vi "校准UI.vi"() -> ()   [LabVIEW 2016, in "斯坦道多参数.lvlib"]
uses:
  <vilib>/Utility/miscctls.llb/LVPointTypeDef.ctl
  <vilib>/Utility/miscctls.llb/LVPositionTypeDef.ctl
  <vilib>/ptbypt/NI_PtbyPt.lvlib
panel:
  out "溶解氧浓度值":dbl=25.0 caption="检测值：" format="%#.2f mg/L"
  out "电极状态标志":u16
  in  "恢复出厂":bool
  in  "电极系数面板":enum32{"选项卡 1"}(tab)
  out "B":dbl=25.0 caption="电极零点：" format="%#.6f"
  out "K":dbl=25.0 caption="电极系数：" format="%#.6f"
  in  "测试参数面板":enum32{"选项卡 1"}(tab)
  in  "自动盐度补偿":bool caption="自动盐度补偿："
  in  "偏移修正值":dbl=25.0 caption="偏移修正值：" format="%#_6f"
  in  "滤波次数":dbl=25.0 caption="滤波次数：" format="%#_6f"
  in  "测量量程":u16(ring)=1 caption="测量量程："
  in  "盐度":dbl=25.0 caption="盐度：" format="%#_6f"
  in  "大气压力":dbl=25.0 caption="大气压力：" format="%#_6f"
  in  "温度系数":dbl=25.0 caption="温度系数：" format="%#6.f"
  out "信号值":dbl=25.0 caption="信号值：" format="%#.2f"
  out "检测值":dbl=25.0 caption="检测值：" format="%#.2f"
  out "序列号":string caption="序列号："
  in  "选项卡控件 3":enum32{"选项卡 1"}(tab)
  in  "清扫间隔":u16=25 caption="清扫间隔："
  in  "清扫次数":u16=25 caption="清扫次数："
  in  "清洗":bool caption="探头清洗："
  in  "清扫模式":u16(ring)=1 caption="清扫模式：" items=["自动", "手动"]
  in  "选项卡控件 2":enum32{"选项卡 1"}(tab)
  in  "实际温度":dbl=25.0 caption="实际温度：" format="%.2f ℃"
  out "当前温度":dbl caption="当前温度：" format="%.2f ℃"
  in  "校准温度":bool
  in  "选项卡控件":enum32{"选项卡 1"}(tab)
  in  "第三点确认校准":bool
  in  "第二点确认校准":bool
  in  "标液一":cluster{"标准值":dbl, "检测值":dbl, "原始值":dbl} caption="标液一：" {"原始值" format="%#_6f"; "检测值" format="%#_6f"; "标准值" format="%#.6f"}
  in  "标液二":cluster{"标准值":dbl, "检测值":dbl, "原始值":dbl} caption="标液二：" {"原始值" format="%#_6f"; "检测值" format="%#_6f"; "标准值" format="%#.6f"}
  in  "标液三":cluster{"标准值":dbl, "检测值":dbl, "原始值":dbl} caption="标液三：" {"原始值" format="%#_6f"; "检测值" format="%#_6f"; "标准值" format="%#.6f"}
  in  "标液一开始校准":bool
  in  "第一点确认校准":bool
  in  "标液二开始校准":bool
  in  "标液三开始校准":bool
  in  "显示曲线":bool
  in  "校准记录":string="校准记录\n---------------------------------------------\n序列号：\n温度值：\n标准值：\n检测值：\n原始值：\n校准时间："
  in  "校准方式":u16(ring)=1 caption="校准方式：" items=["单点校准", "两点校准", "三点校准"]
  in  "校准参数":u16(ring) caption="校准参数：" items=["pH", "DO", "浊度", "电导率"]
  # "检测值"
  # "信号值"
  # "标准值"
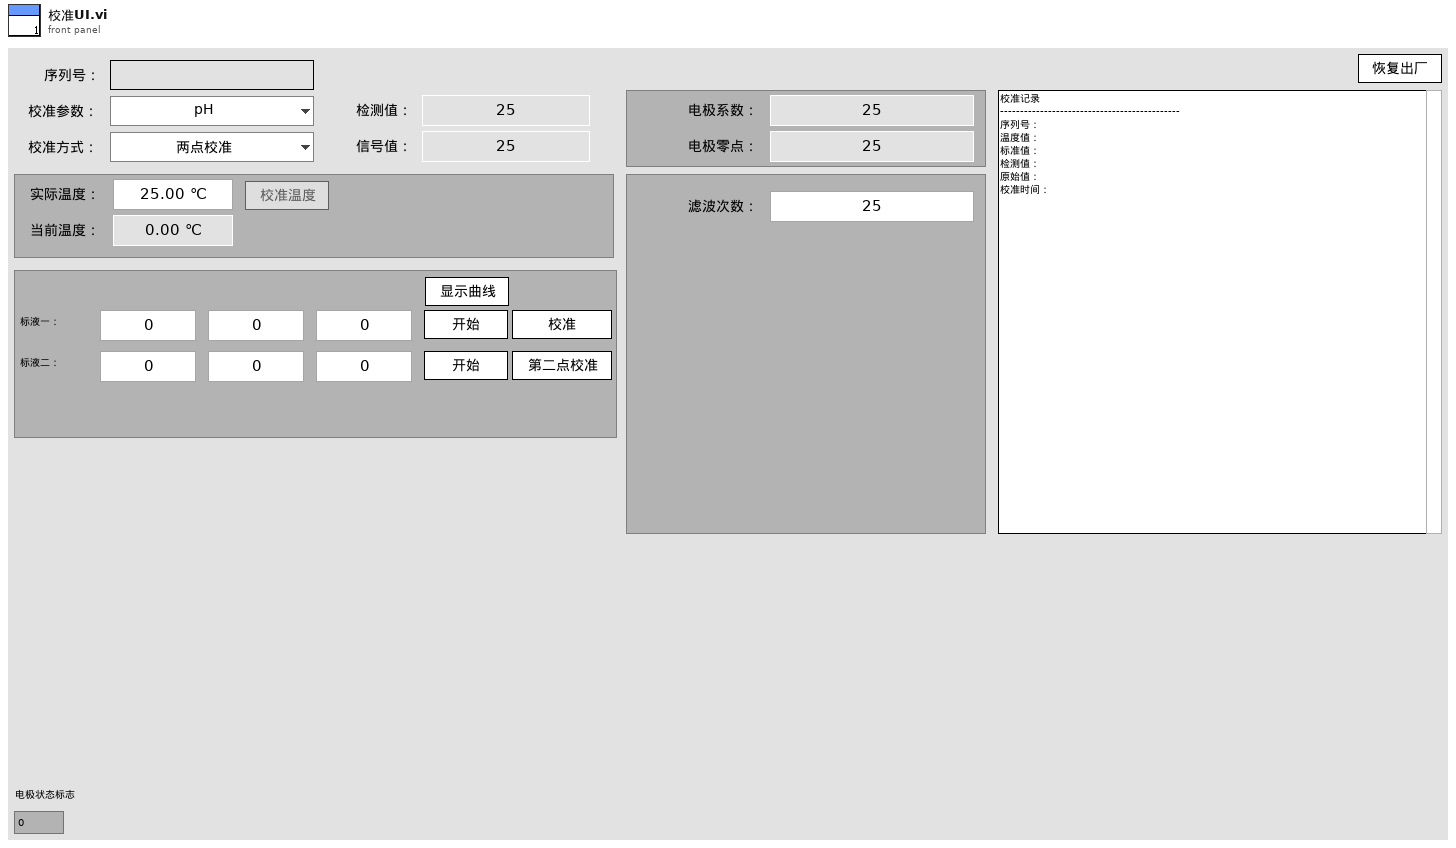
[diagram p1: front panel]
types:
  T1 = typedef "LVPointTypeDef.ctl" = cluster{"Horizontal":i16, "Vertical":i16}
  T2 = cluster{"ph":bool, "DO":bool, "Cond":bool, "Turb":bool, "叶绿素a":bool, "藻密度":bool, "ORP":bool, "COD":bool, "DO2":bool}
  T3 = typedef "LVStringsAndValuesArrayTypeDef_U16.ctl" = cluster{"String":string, "Value":u16}[]
  T4 = enum8{"Enabled", "Disabled", "Disabled and Grayed Out"}
  T5 = typedef "LVPositionTypeDef.ctl" = cluster{"Left":i32, "Top":i32}
  T6 = cluster{"pH":u32, "DO":u32, "Cond":u32, "Turb":u32, "叶绿素a":u32, "藻密度":u32, "ORP":u32, "COD":u32}
  T7 = cluster{"电极状态标志":u16, "电极型号标志":u16, "酸碱度测量值":sgl, "温度测量值":sgl, "酸碱度信号值":sgl, "温度信号值":sgl, "酸碱度偏移修正值":sgl, "温度偏移修正值":sgl, "手动温度补偿值":sgl, "酸碱度电极零点":sgl, "酸碱度电极斜率":sgl, "第1点标准值记录":sgl, "第1点信号值记录":sgl, "第1点温度值记录":sgl, "第2点标准值记录":sgl, "第2点信号值记录":sgl, "第2点温度值记录":sgl, "命令滤波设定":u16, "温度模式":enum16{"ATC", "MTC"}, "生产批次":u16, "电极序号":u16, "串口地址":u16, "串口波特率":enum16{"9600", "19200", "115200"}, "串口校验位":enum16{"NONE", "ODD", "EVEN"}, "串口停止位":enum16{"1bit", "2bit"}, "第一点标准值":sgl, "第二点标准值":sgl}
  T8 = cluster{"报警码":u16, "溶解氧数值（mg/L）":sgl, "溶解氧数据（%）":sgl, "温度数据":sgl, "溶解氧原始信号 nA":sgl, "大气压力":sgl, "盐度":sgl, "0X0009_NC":string, "产品名称":string, "序列号":string, "硬件版本":string, "软件版本":string, "通讯地址":u16, "波特率":u16, "设备类型":u16, "0X0026_NC":string, "第一点原始数据":sgl, "第一点校准数据":sgl, "第二点原始数据":sgl, "第二点校准数据":sgl, "探头校准命令":u16, "温度校准参数":sgl, "温度校准命令":u16}
  T9 = cluster{"电极状态标志":u16, "电极型号标志":u16, "溶解氧测量值":sgl, "温度测量值":sgl, "溶解氧饱和度值":sgl, "盐度补偿值":sgl, "大气压补偿值":sgl, "溶解氧偏移修正值":sgl, "温度偏移修正值":sgl, "手动温度补偿值":sgl, "溶解氧电极零点":sgl, "溶解氧电极斜率":sgl, "第1点标准值记录":sgl, "第1点信号值记录":sgl, "第1点温度值记录":sgl, "第2点标准值记录":sgl, "第2点信号值记录":sgl, "第2点温度值记录":sgl, "命令滤波设定":u16, "温度模式":enum16{"ATC", "MTC"}, "生产批次":u16, "电极序号":u16, "串口地址":u16, "串口波特率":enum16{"9600", "19200", "115200"}, "串口校验位":enum16{"NONE", "ODD", "EVEN"}, "串口停止位":enum16{"1bit", "2bit"}, "第一点标准值":sgl, "第二点标准值":sgl}
  T10 = cluster{"电极状态标志":u16, "电极型号标志":u16, "浊度测量值":sgl, "温度测量值":sgl, "浊度信号值":sgl, "浊度偏移修正值":sgl, "温度偏移修正值":sgl, "手动温度补偿值":sgl, "浊度电极零点":sgl, "浊度电极斜率":sgl, "清洁周期":u16, "命令滤波设定":u16, "温度模式":enum16{"ATC", "MTC"}, "生产批次":u16, "电极序号":u16, "串口地址":u16, "串口波特率":enum16{"9600", "19200", "115200"}, "串口校验位":enum16{"NONE", "ODD", "EVEN"}, "串口停止位":enum16{"1bit", "2bit"}, "第一点标准值":sgl, "第二点标准值":sgl, "第三点标准值":sgl}
  T11 = cluster{"报警码":u16, "浊度数值 NTU":sgl, "温度数据":sgl, "原始光强数值":u16, "量程":u16, "平均次数":u16, "清扫模式":u16, "清扫次数":u16, "清扫间隔分钟":u16, "0X000B_NC":string, "产品名称":string, "序列号":string, "硬件版本":string, "软件版本":string, "通讯地址":u16, "波特率":u16, "设备类型":u16, "0X0026_NC":string, "校准量程":u16, "第一点原始光强":u16, "第一点校准数据":sgl, "第二点原始光强":u16, "第二点校准数据":sgl, "第三点原始光强":u16, "第三点校准数据":sgl, "探头校准命令":u16, "温度校准参数":sgl, "温度校准命令":u16}
  T12 = cluster{"电极状态标志":u16, "电极型号标志":u16, "电导率测量值":sgl, "温度测量值":sgl, "电导率信号值":sgl, "温度信号值":sgl, "温度补偿系数":sgl, "电导率偏移修正值":sgl, "温度偏移修正值":sgl, "手动温度补偿值":sgl, "电导率电极零点":sgl, "电导率电极斜率":sgl, "命令滤波设定":u16, "温度模式":enum16{"ATC", "MTC"}, "生产批次":u16, "电极序号":u16, "串口地址":u16, "串口波特率":enum16{"9600", "19200", "115200"}, "串口校验位":enum16{"NONE", "ODD", "EVEN"}, "串口停止位":enum16{"1bit", "2bit"}, "第一点标准值":sgl, "第二点标准值":sgl}
  T13 = cluster{"报警码":u16, "叶绿素a":sgl, "温度数据":sgl, "原始光强数值":u16, "量程":u16, "平均次数":u16, "清扫模式":u16, "清扫次数":u16, "清扫间隔分钟":u16, "0X000B_NC":string, "产品名称":string, "序列号":string, "硬件版本":string, "软件版本":string, "通讯地址":u16, "波特率":u16, "设备类型":u16, "0X0026_NC":string, "校准量程":u16, "第一点原始光强":u16, "第一点校准数据":sgl, "第二点原始光强":u16, "第二点校准数据":sgl, "第三点原始光强":u16, "第三点校准数据":sgl, "探头校准命令":u16, "温度校准参数":sgl, "温度校准命令":u16}
  T14 = cluster{"报警码":u16, "蓝绿藻":sgl, "温度数据":sgl, "原始光强数值":u16, "量程":u16, "平均次数":u16, "清扫模式":u16, "清扫次数":u16, "清扫间隔分钟":u16, "0X000B_NC":string, "产品名称":string, "序列号":string, "硬件版本":string, "软件版本":string, "通讯地址":u16, "波特率":u16, "设备类型":u16, "0X0026_NC":string, "校准量程":u16, "第一点原始光强":u16, "第一点校准数据":sgl, "第二点原始光强":u16, "第二点校准数据":sgl, "第三点原始光强":u16, "第三点校准数据":sgl, "探头校准命令":u16, "温度校准参数":sgl, "温度校准命令":u16}
  T15 = cluster{"电极状态标志":u16, "电极型号标志":u16, "测量值":sgl, "温度测量值":sgl, "信号值":sgl, "温度信号值":sgl, "000AH_NC":sgl, "偏移修正值":sgl, "温度偏移修正值":sgl, "手动温度补偿值":sgl, "命令滤波设定":u16, "温度模式":enum16{"ATC", "MTC"}, "生产批次":u16, "传感器序号":u16, "串口地址":u16, "串口波特率":enum16{"9600", "19200", "115200"}, "串口校验位":enum16{"NONE", "ODD", "EVEN"}, "串口停止位":enum16{"1bit", "2bit"}}
  T16 = enum16{"null", "pH", "DO", "浊度", "电导率", "叶绿素a", "藻密度"}
  T17 = cluster{"禁用":enum8{"Enabled", "Disabled", "Disabled and Grayed Out"}, "禁用 2":enum8{"Enabled", "Disabled", "Disabled and Grayed Out"}, "禁用 3":enum8{"Enabled", "Disabled", "Disabled and Grayed Out"}}
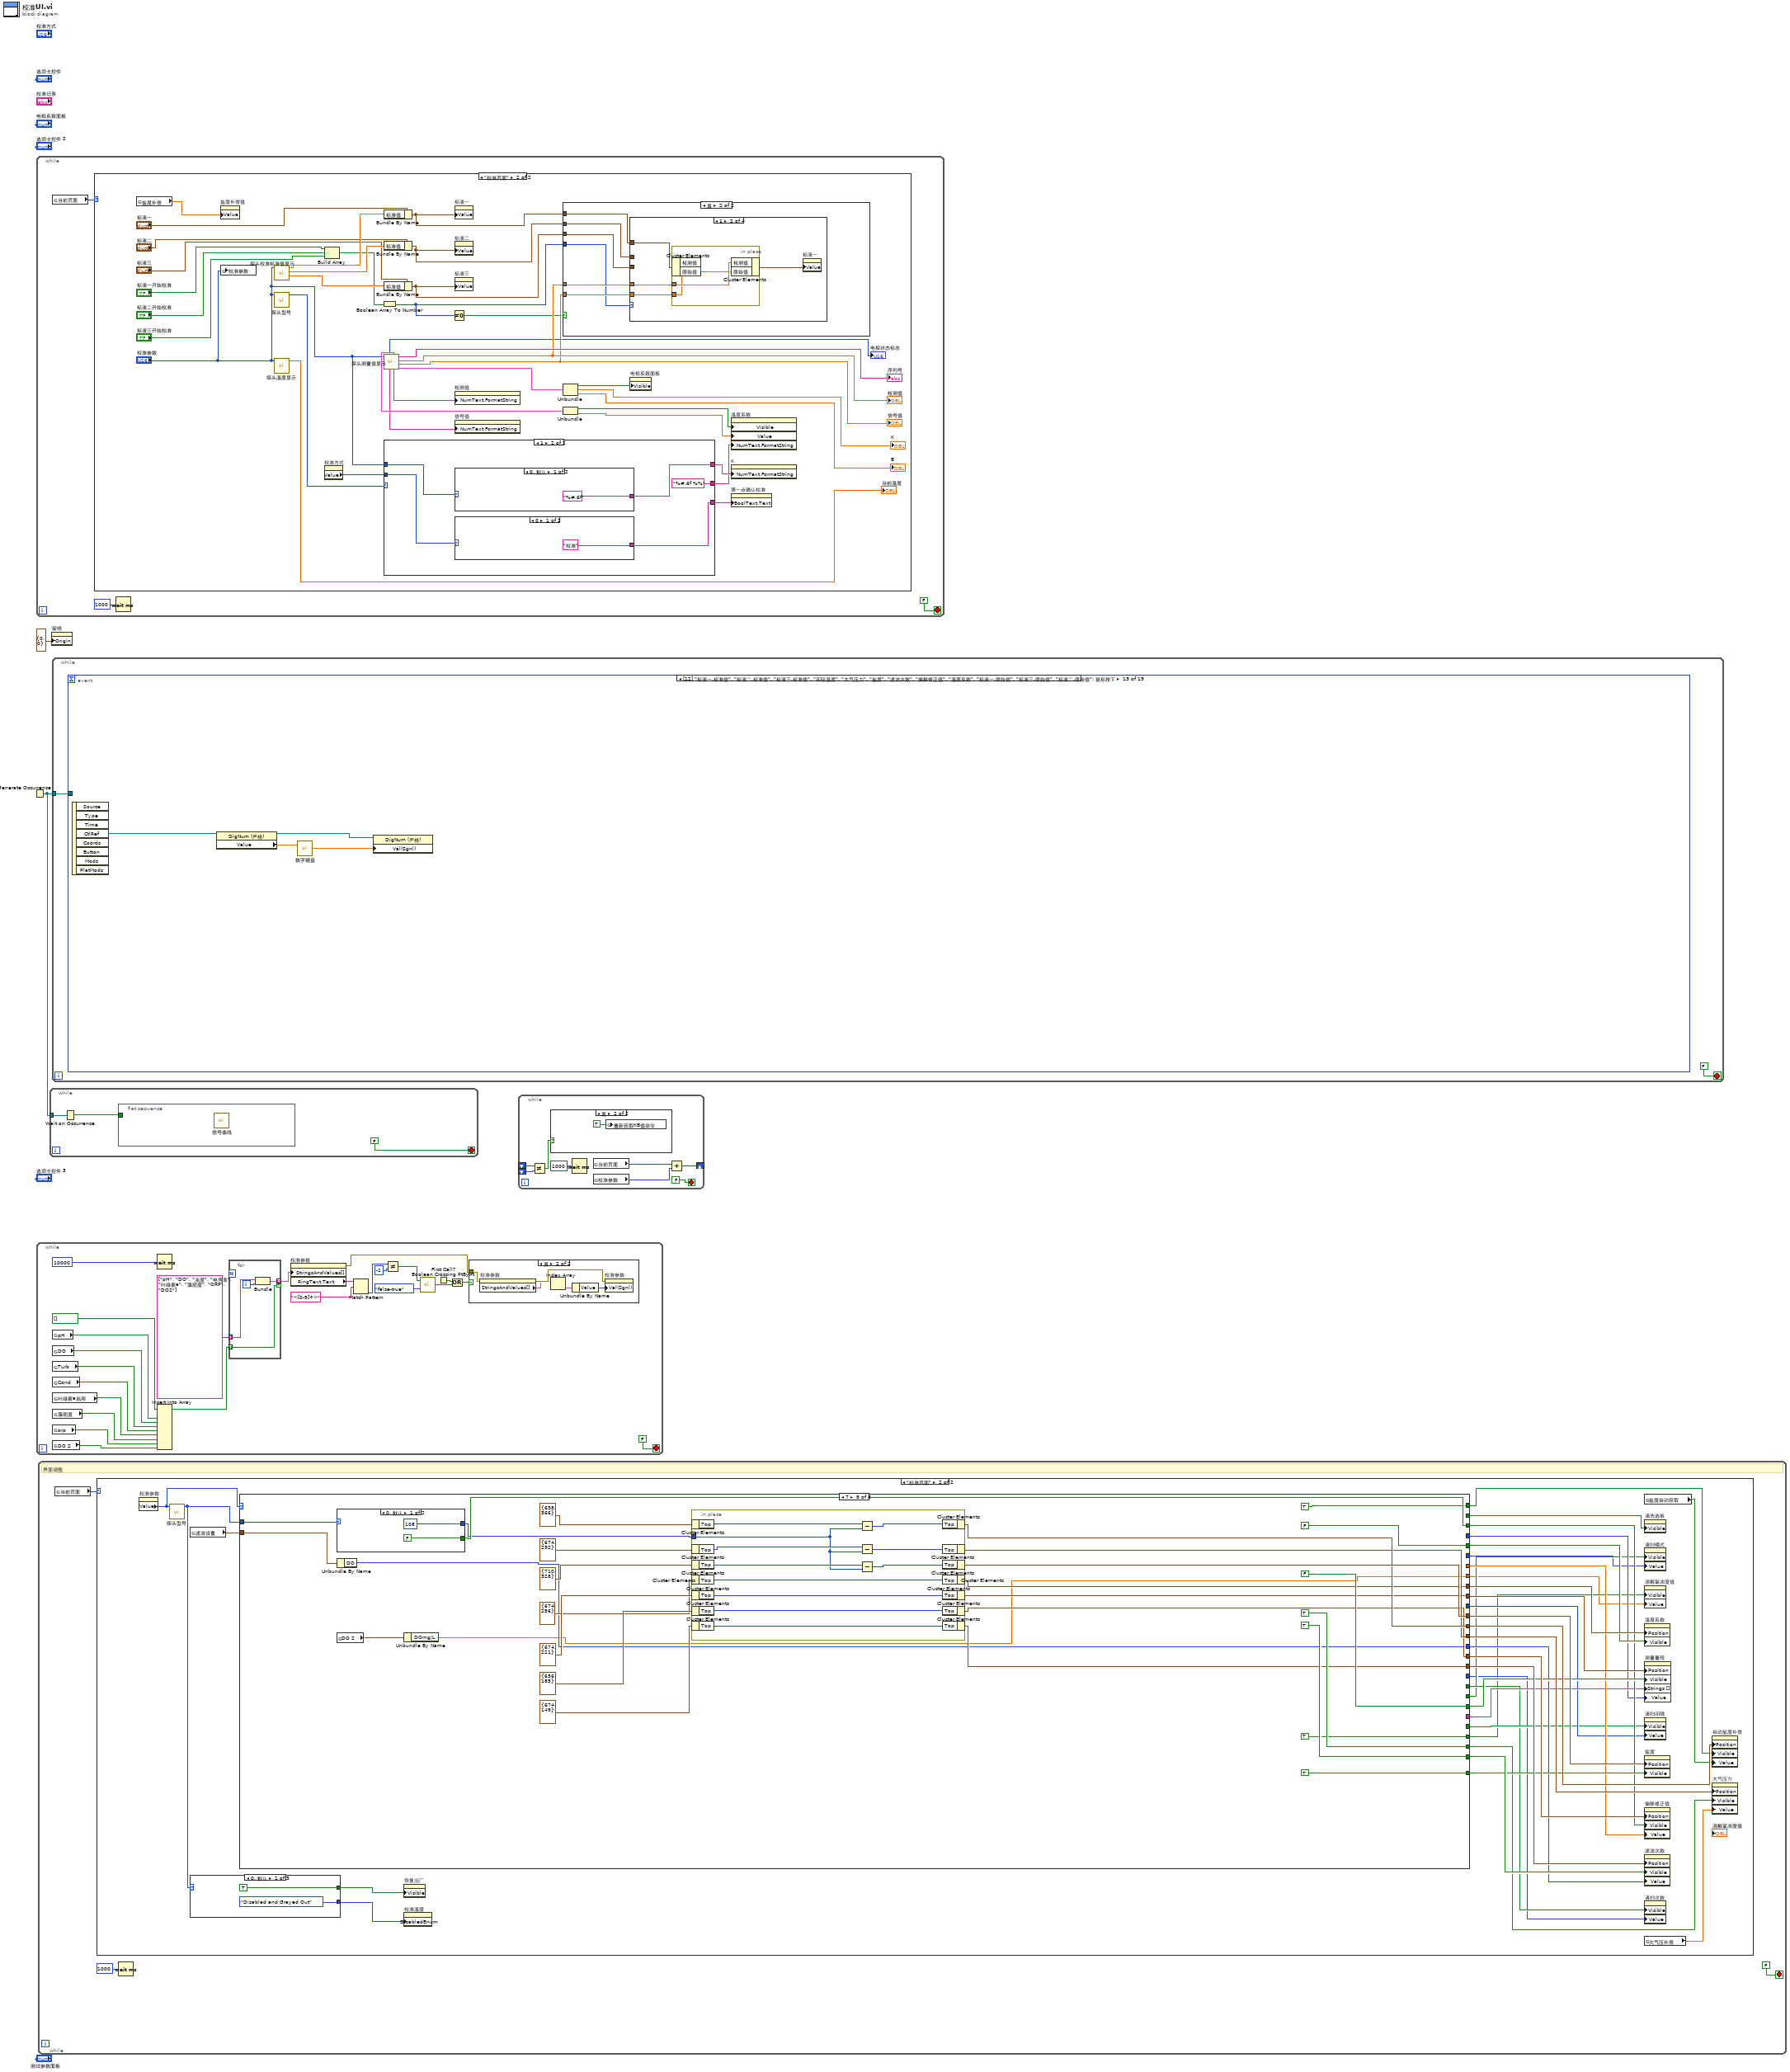
[diagram p0: block diagram]
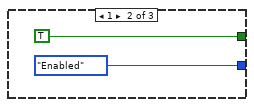
[diagram p4: hidden frame]
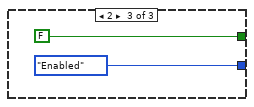
[diagram p5: hidden frame]
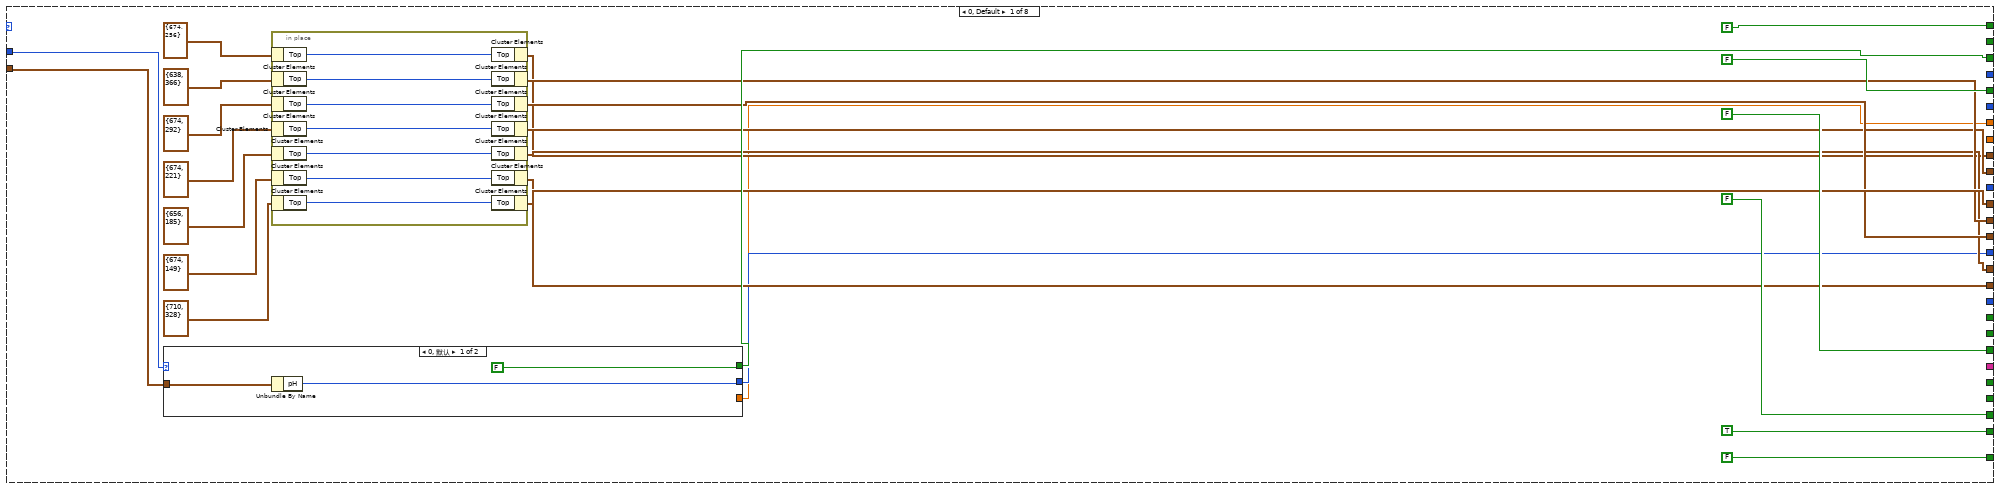
[diagram p6: hidden frame]
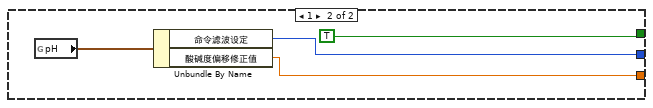
[diagram p7: hidden frame]
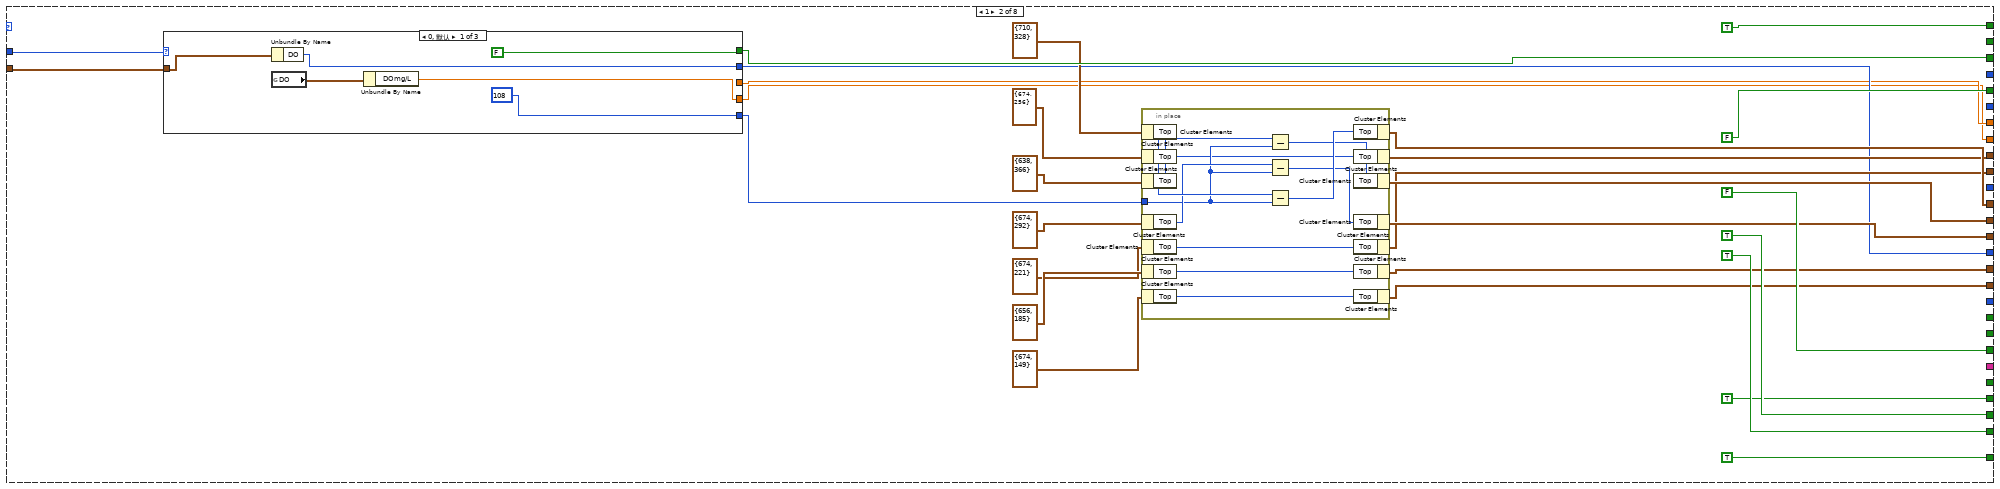
[diagram p8: hidden frame]
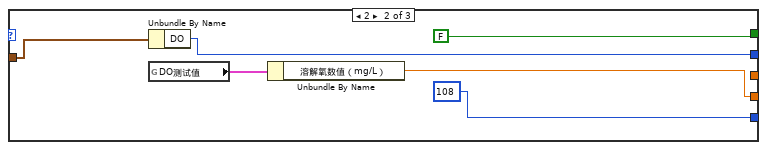
[diagram p9: hidden frame]
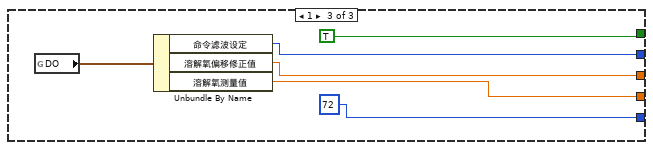
[diagram p10: hidden frame]
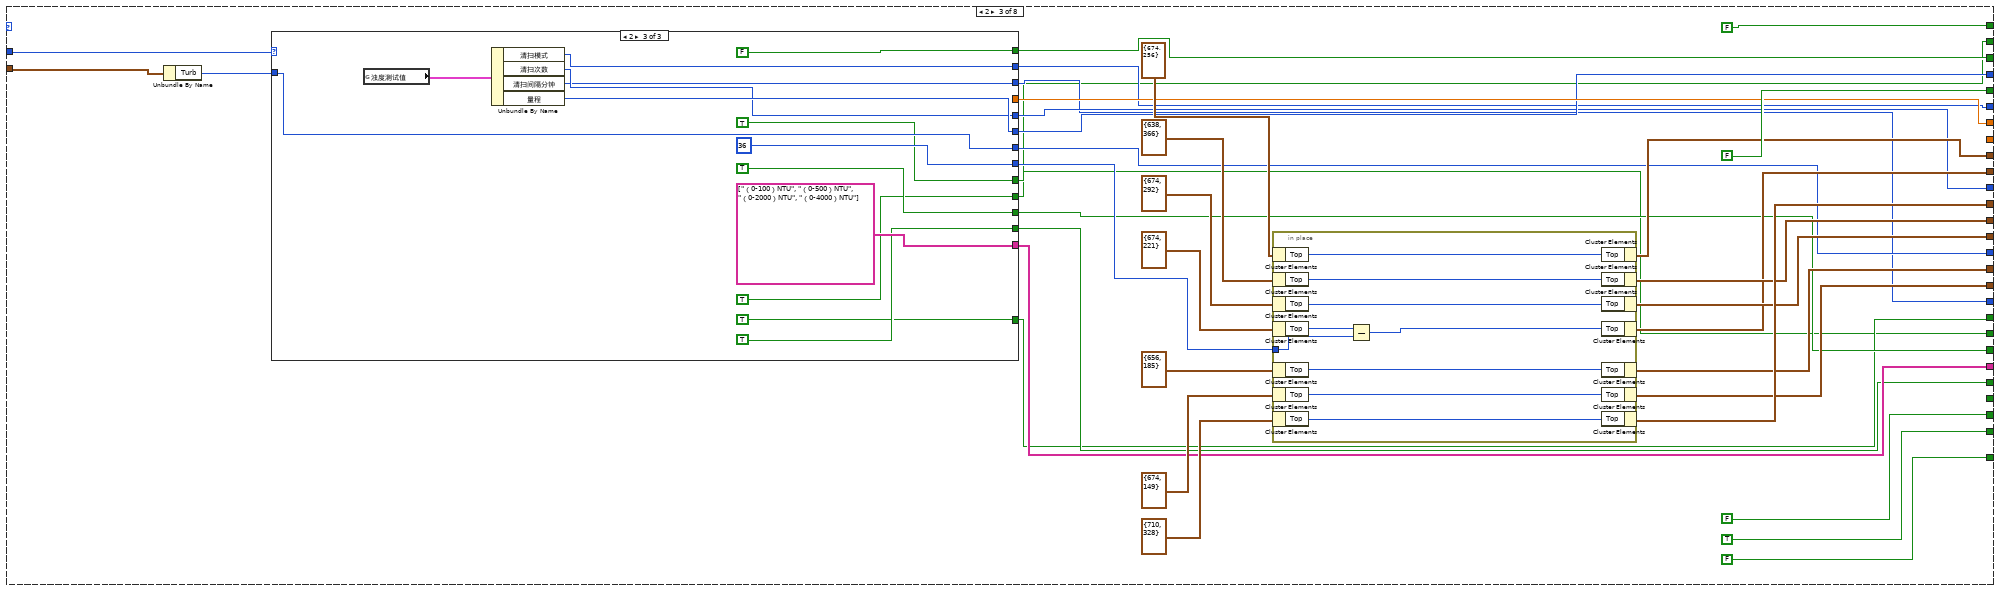
[diagram p11: hidden frame]
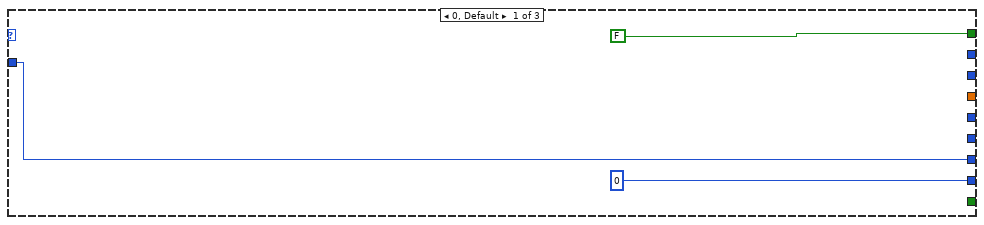
[diagram p12: hidden frame]
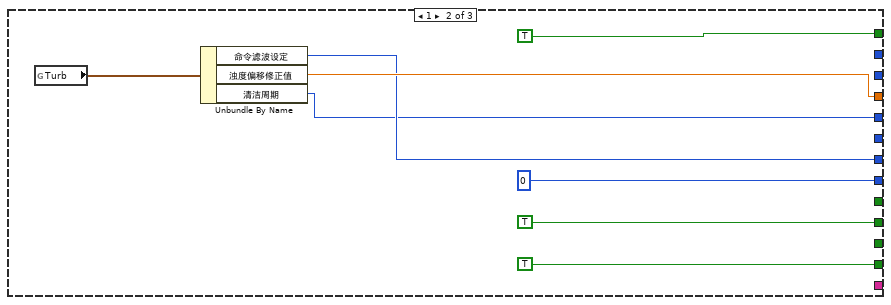
[diagram p13: hidden frame]
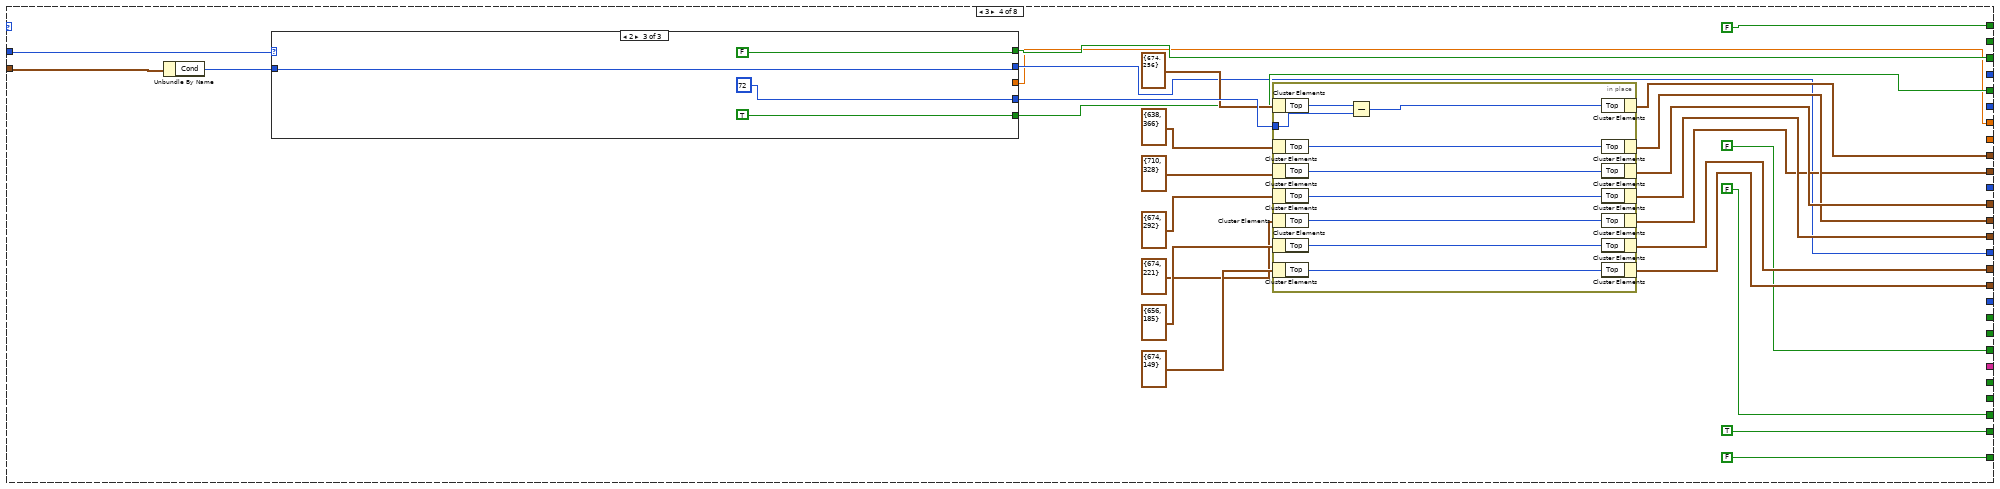
[diagram p14: hidden frame]
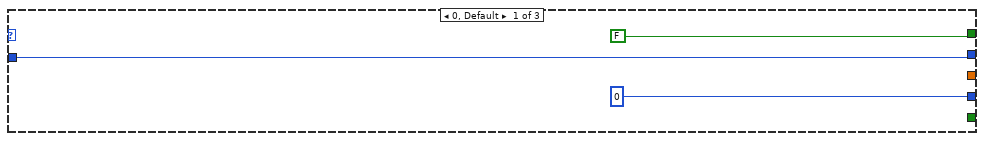
[diagram p15: hidden frame]
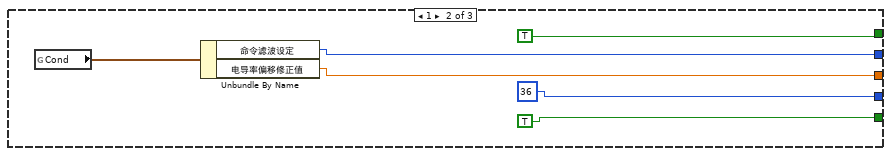
[diagram p16: hidden frame]
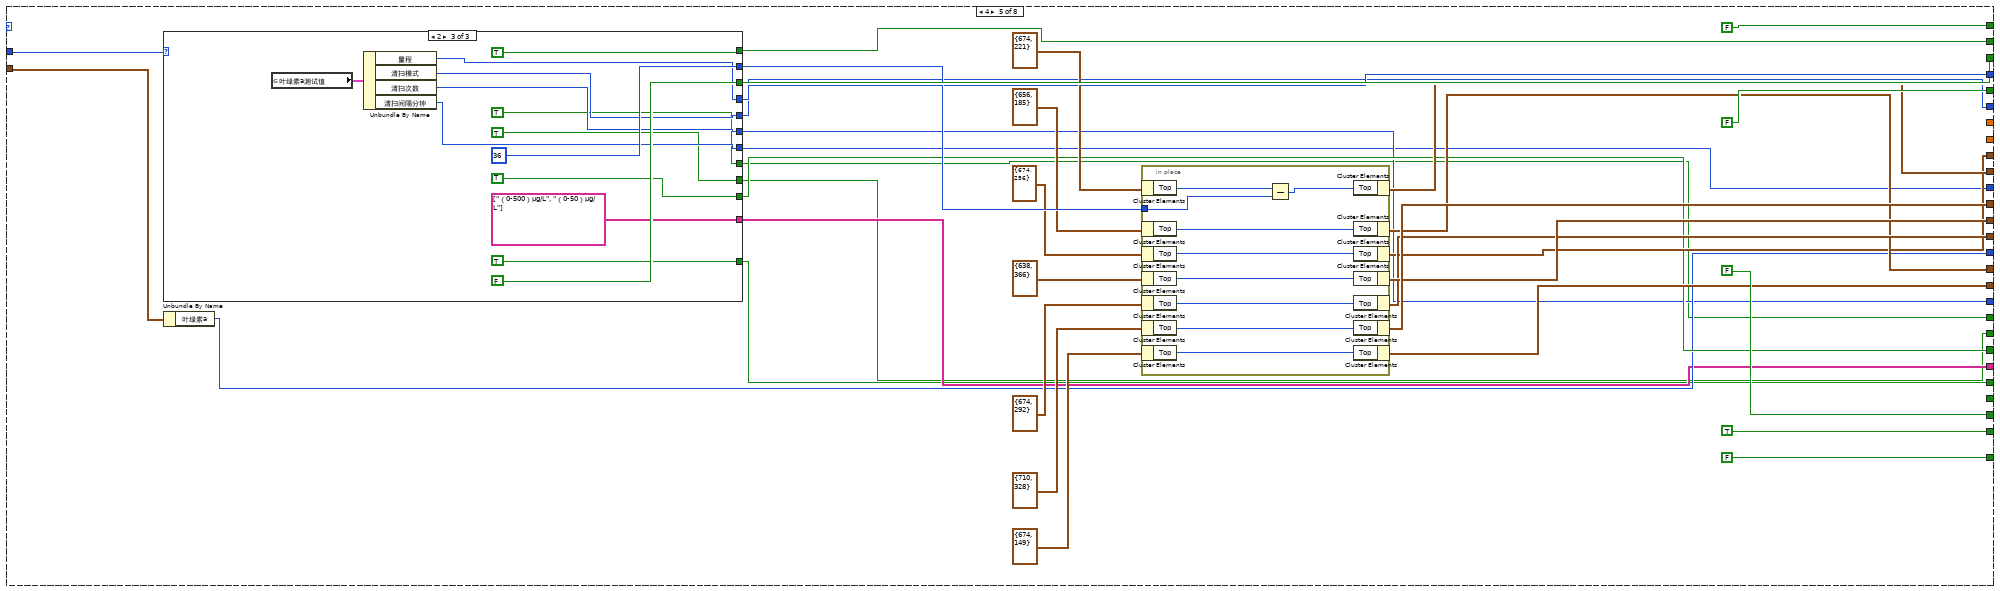
[diagram p17: hidden frame]
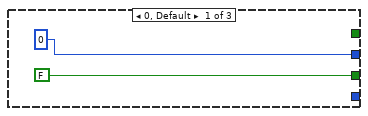
[diagram p18: hidden frame]
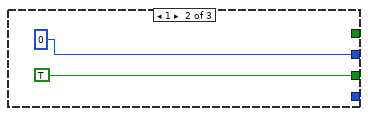
[diagram p19: hidden frame]
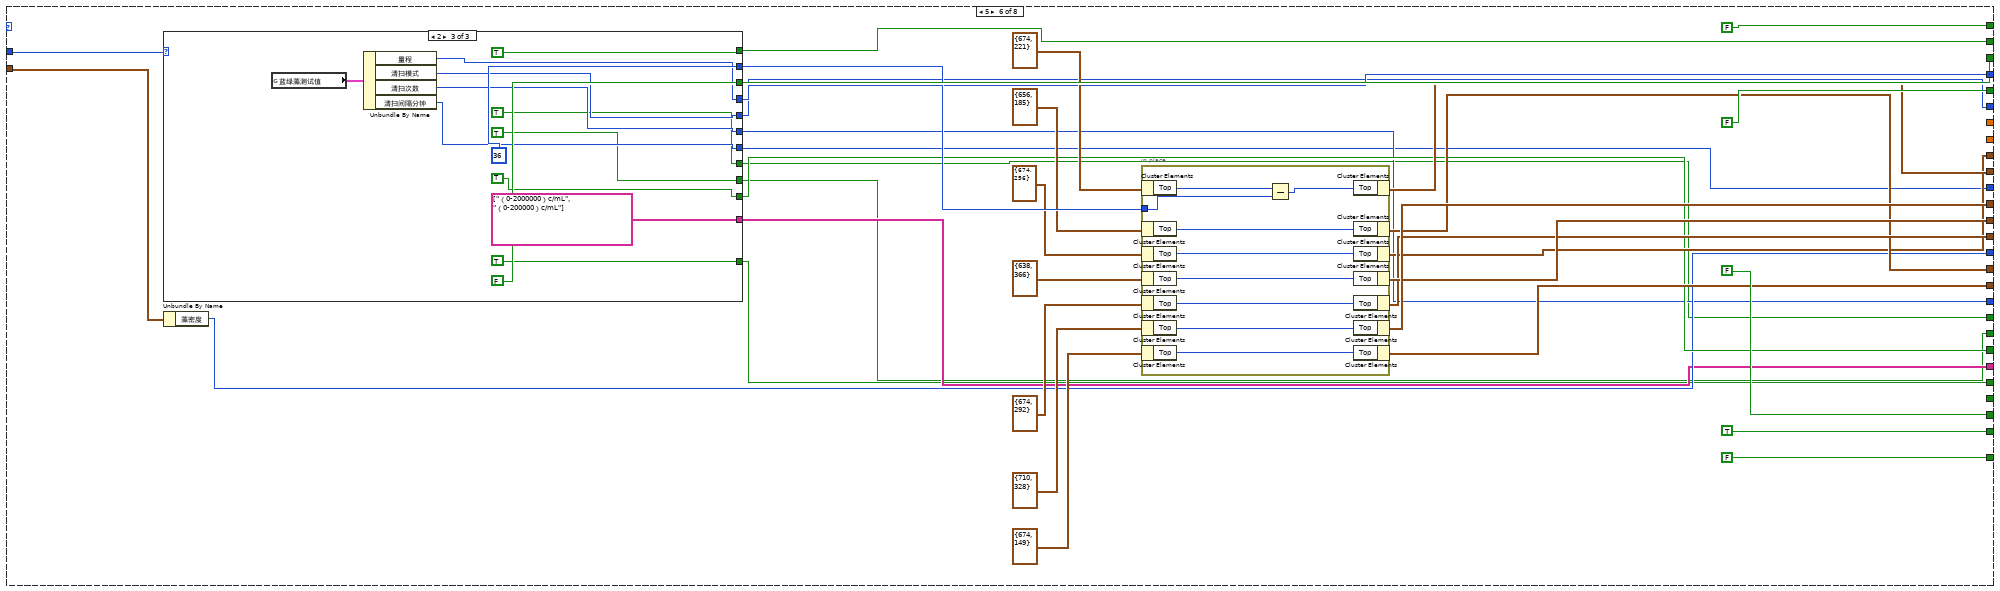
[diagram p20: hidden frame]
diagram:
  n1 = Generate Occurrence() -> (w1:refnum<k4>)
  n2 = while {
    stop <- FALSE stop-if-true
    n3 = global read "多参数全局变量.vi" "当前页面"() -> (w3:enum16{"主页面", "参数页面", "校准页面"})
    n4 = case shown="\"校准页面\"" w3 {
      frame "主页面", Default {
        n5 = global write "多参数全局变量.vi" "校准运行状态"(T2 {"ph"=FALSE, "DO"=FALSE, "Cond"=FALSE, "Turb"=FALSE, "叶绿素a"=FALSE, "藻密度"=FALSE, "ORP"=FALSE, "COD"=FALSE, "DO2"=FALSE} ("校准运行状态")) -> ()
      }
      frame "校准页面" {
        n6 = global read "断电保存变量.vi" "盐度补偿"() -> (w29:dbl)
        n7 = property on="盐度补偿值" class="DigNum (严格)"("Value"=w29) -> ()  [unwired: 2 in, 2 out]
        n8 = global write "多参数全局变量.vi" "校准参数"("校准参数") -> ()
        n9 = call "探头校准标准值显示.vi"("校准参数"="校准参数") -> ("标液三"=w42:sgl, "标液二"=w41:sgl, "标液一"=w40:sgl)  [unwired: 8 in]
        n10 = call "探头型号.vi"("校准参数"="校准参数") -> ("探头型号"=w24:u16)  [unwired: 8 in, 2 out]
        n11 = call "探头温度显示.vi"("校准参数"="校准参数") -> ("温度数据"=→"当前温度":sgl)  [unwired: 9 in, 1 out]
        n12 = Build Array("标液一开始校准", "标液二开始校准", "标液三开始校准") -> (w10:bool[])
        n13 = property on="校准方式" class="Ring (严格)"() -> ("Value"=w22:u16)  [unwired: 2 in, 2 out]
        n14 = Boolean Array To Number(Boolean array=w10) -> (number=w8:u32)
        n15 = Bundle By Name(cluster="标液一", "标准值"=w40) -> (w36:cluster{"标准值":dbl, "检测值":dbl, "原始值":dbl})
        n16 = Bundle By Name(cluster="标液二", "标准值"=w41) -> (w35:cluster{"标准值":dbl, "检测值":dbl, "原始值":dbl})
        n17 = Bundle By Name(cluster="标液三", "标准值"=w42) -> (w34:cluster{"标准值":dbl, "检测值":dbl, "原始值":dbl})
        n18 = call "探头测量值显示.vi"("校准参数"="校准参数") -> ("线性系数"=w28:cluster{bool, "K":sgl, "B":sgl}, "信号值"=w30:sgl, "检测值"=w31:sgl, "序列号"=→"序列号":string, "检测值.格式字符串"=w21:string, "温度补偿系数"=w20:cluster{bool, "温度补偿系数":sgl}, "信号值.格式字符串"=w16:string, "电极状态标志"=→"电极状态标志":u16)  [unwired: 3 in]
        "检测值" <- w31
        "信号值" <- w30
        n19 = case shown="1" w24 {
          tunnel: ["校准" w50] -> w23
          tunnel: w22 -> [_ w49]
          tunnel: "校准参数" -> [_ w48]
          tunnel: ["%#.6f" ("数值文本.格式字符串") w47] -> w15
          tunnel: ["%#.6f" ("数值文本.格式字符串") "%#.6f %%" ("数值文本.格式字符串")] -> w14
          frame 0, Default {
          }
          frame 1 {
            n20 = case shown="0, 默认" w48 {
              tunnel: ["%#.6f" ("数值文本.格式字符串") "%#.6f (1/cm)" ("数值文本.格式字符串")] -> w47
              frame 0, Default {
              }
              frame 3 {
              }
            }
            n21 = case shown="0" w49 {
              tunnel: ["校准" "第一点校准"] -> w50
              frame 0 {
              }
              frame 1, Default {
              }
            }
          }
        }
        n22 = Not Equal To 0?(x=w8) -> (x != 0?=w9:bool)
        n23 = property on="标液一" class="Clust (严格)"("Value"=w36) -> ()  [unwired: 2 in, 2 out]
        n24 = property on="标液二" class="Clust (严格)"("Value"=w35) -> ()  [unwired: 2 in, 2 out]
        n25 = property on="标液三" class="Clust (严格)"("Value"=w34) -> ()  [unwired: 2 in, 2 out]
        n26 = property on="检测值" class="DigNum (严格)"("NumText.FormatString"=w21) -> ()  [unwired: 2 in, 2 out]
        n27 = property on="信号值" class="DigNum (严格)"("NumText.FormatString"=w16) -> ()  [unwired: 2 in, 2 out]
        n28 = case shown="真" w9 {
          tunnel: w36 -> [_ w60]
          tunnel: w35 -> [_ w59]
          tunnel: w34 -> [_ w58]
          tunnel: w30 -> [_ w57]
          tunnel: w31 -> [_ w56]
          tunnel: w8 -> [_ w55]
          frame False {
          }
          frame True {
            n29 = case shown="1" w55 {
              tunnel: w56 -> [_ w63 w70 w76]
              tunnel: w57 -> [_ w62 w69 w75]
              tunnel: w60 -> [_ w64 _ _]
              tunnel: w59 -> [_ _ w67 _]
              tunnel: w58 -> [_ _ _ w73]
              frame Default {
              }
              frame 1 {
                n30 = in-place {
                  in-place-border: w63 -> [w66]
                  in-place-border: w62 -> [w65]
                  n31 = in-place-cluster #1(w64) -> ()  [unwired: 2 out]
                  n32 = in-place-cluster #1("检测值"=w66, "原始值"=w65) -> (w61:cluster{"标准值":dbl, "检测值":dbl, "原始值":dbl})
                }
                n33 = property on="标液一" class="Clust (严格)"("Value"=w61) -> ()  [unwired: 2 in, 2 out]
              }
              frame 2 {
                n34 = in-place {
                  in-place-border: w70 -> [w72]
                  in-place-border: w69 -> [w71]
                  n35 = in-place-cluster #2(w67) -> ()  [unwired: 2 out]
                  n36 = in-place-cluster #2("检测值"=w72, "原始值"=w71) -> (w68:cluster{"标准值":dbl, "检测值":dbl, "原始值":dbl})
                }
                n37 = property on="标液二" class="Clust (严格)"("Value"=w68) -> ()  [unwired: 2 in, 2 out]
              }
              frame 4 {
                n38 = in-place {
                  in-place-border: w76 -> [w78]
                  in-place-border: w75 -> [w77]
                  n39 = in-place-cluster #3(w73) -> ()  [unwired: 2 out]
                  n40 = in-place-cluster #3("检测值"=w78, "原始值"=w77) -> (w74:cluster{"标准值":dbl, "检测值":dbl, "原始值":dbl})
                }
                n41 = property on="标液三" class="Clust (严格)"("Value"=w74) -> ()  [unwired: 2 in, 2 out]
              }
            }
          }
        }
        n42 = Unbundle(w28) -> (w27:bool, "K"=→"K":sgl, "B"=→"B":sgl)
        n43 = Unbundle(w20) -> (w19:bool, "温度补偿系数"=w18:sgl)
        n44 = property on="电极系数面板" class="TabCtl (严格)"("Visible"=w27) -> ()  [unwired: 2 in, 2 out]
        n45 = property on="温度系数" class="DigNum (严格)"("Visible"=w19, "Value"=w18, "NumText.FormatString"=w14) -> ()  [unwired: 2 in, 2 out]
        n46 = property on="K" class="DigNum (严格)"("NumText.FormatString"=w15) -> ()  [unwired: 2 in, 2 out]
        n47 = property on="第一点确认校准" class="Bool"("BoolText.Text"=w23) -> ()  [unwired: 2 in, 2 out]
      }
    }
    n48 = Wait (ms)(milliseconds to wait=u32 1000 ("等待时间（毫秒）")) -> ()  [unwired: 1 out]
  }
  n49 = while {
    stop <- FALSE stop-if-true
    n50 = global read "断电保存变量.vi" "pH"() -> (w102:bool)
    n51 = global read "断电保存变量.vi" "DO"() -> (w100:bool)
    n52 = global read "断电保存变量.vi" "Turb"() -> (w99:bool)
    n53 = global read "断电保存变量.vi" "Cond"() -> (w98:bool)
    n54 = global read "断电保存变量.vi" "叶绿素a启用"() -> (w97:bool)
    n55 = global read "断电保存变量.vi" "藻密度"() -> (w96:bool)
    n56 = global read "断电保存变量.vi" "orp"() -> (w95:bool)
    n57 = global read "断电保存变量.vi" "DO 2"() -> (w94:bool)
    n58 = Wait (ms)(milliseconds to wait=u32 10000 ("等待时间（毫秒）")) -> ()  [unwired: 1 out]
    n59 = Insert Into Array(array=bool[] [] ("数组"), new element #1=w102, new element #2=w100, new element #3=w99, new element #4=w98, new element #5=w97, new element #6=w96, new element #7=w95, new element #8=w94) -> (w91:bool[])  [unwired: 1 in]
    n60 = for {
      tunnel: w91 -> [w108] mode=indexing
      tunnel: string[] ["pH", "DO", "浊度", "电导率", "叶绿素a", "藻密度", "ORP", "DO2"] ("字符串[]") -> [w110] mode=indexing
      tunnel: [w109] -> w88 mode=indexing if=w108
      i -> [w111]
      n61 = Bundle(w110, w111) -> (w109:cluster{string, i32})  [unwired: 1 in]
    }
    n62 = property on="校准参数" class="Ring (严格)"("StringsAndValues[]"=w88) -> (error out=w89:errorcluster, "RingText.Text"=w87:string)  [unwired: 2 in, 1 out]
    n63 = Match Pattern(string=w87, regular expression="<[0-9]+>" ("正则表达式")) -> (offset past match=w85:i32)  [unwired: 1 in, 3 out]
    n64 = Not Equal?(x=w85, y=-1) -> (x != y?=w83:bool)
    n65 = call <vilib>:"Boolean Crossing PtByPt.vi"("direction"=enum16{"either", "false-true", "true-false"}."false-true", "input"=w83) -> ("crossing"=w80:bool)  [unwired: 1 in]
    n66 = First Call?() -> (First Call?: T/F=w81:bool)
    n67 = Or(x=w81, y=w80) -> (x .or. y?=w82:bool)
    n68 = case shown="真" w82 {
      tunnel: w89 -> [_ w107]
      frame False {
      }
      frame True {
        n69 = property on="校准参数" class="Ring (严格)"(error in=w107) -> (error out=w106:errorcluster, "StringsAndValues[]"=w105:T3)  [unwired: 1 in, 1 out]
        n70 = Index Array(array=w105) -> (element=w104:cluster{"String":string, "Value":u16})  [unwired: 1 in]
        n71 = Unbundle By Name(w104) -> ("Value"=w103:u16)
        n72 = property on="校准参数" class="Ring (严格)"(error in=w106, "Val(Sgnl)"=w103) -> ()  [unwired: 1 in, 2 out]
      }
    }
  }
  n73 = while {
    stop <- FALSE stop-if-true
    # "界面调整"
    n74 = global read "多参数全局变量.vi" "当前页面"() -> (w113:enum16{"主页面", "参数页面", "校准页面"})
    n75 = case shown="\"校准页面\"" w113 {
      frame "主页面", Default {
      }
      frame "校准页面" {
        n76 = property on="校准参数" class="Ring (严格)"() -> ("Value"=w147:u16)  [unwired: 2 in, 2 out]
        n77 = call "探头型号.vi"("校准参数"=w147) -> ("探头型号"=w117:u16)  [unwired: 8 in, 2 out]
        n78 = global read "断电保存变量.vi" "滤波设置"() -> (w129:T6)
        n79 = case shown="0, 默认" w117 {
          tunnel: [TRUE TRUE FALSE] -> w116
          tunnel: [T4."Disabled and Grayed Out" ("禁用") T4."Enabled" ("禁用") T4."Enabled" ("禁用")] -> w115
          frame 0, Default {
          }
          frame 1 {
          }
          frame 2 {
          }
        }
        n80 = case shown="7" w147 {
          tunnel: [w164 w205 w271 w333 w388 w448 w500 w540] -> w148
          tunnel: w117 -> [w172 w214 w280 w342 w397 w457 w508 w549]
          tunnel: [w162 w203 w269 w331 w386 w446 w498 w538] -> w146
          tunnel: [w160 w201 w267 w329 w384 w444 w496 w536] -> w145
          tunnel: [w158 w199 w265 w327 w382 w442 w494 w534] -> w144
          tunnel: [w166 w207 w273 w335 w390 w450 w502 w542] -> w143
          tunnel: [w168 w210 w276 w338 w393 w453 w504 w545] -> w142
          tunnel: [w167 w208 w274 w336 w391 w451 w503 w543] -> w141
          tunnel: [TRUE TRUE TRUE TRUE TRUE TRUE TRUE TRUE] -> w140
          tunnel: [FALSE FALSE w264 FALSE w381 w441 FALSE FALSE] -> w139
          tunnel: [FALSE TRUE FALSE FALSE FALSE FALSE FALSE TRUE] -> w138
          tunnel: [FALSE FALSE FALSE w325 FALSE FALSE FALSE FALSE] -> w137
          tunnel: [w175 w217 w283 w345 w400 w460 w511 w552] -> w136
          tunnel: [FALSE TRUE FALSE FALSE FALSE FALSE FALSE TRUE] -> w135
          tunnel: [FALSE TRUE FALSE FALSE FALSE FALSE FALSE TRUE] -> w134
          tunnel: [w157 w197 w262 w322 w379 w439 w492 w532] -> w131
          tunnel: [w156 w196 w263 w321 _ _ w493 _] -> w130
          tunnel: w129 -> [w155 w198 w261 w324 w380 w440 w491 w533]
          tunnel: [_ _ w259 _ w378 w438 _ _] -> w128
          tunnel: [_ _ w258 _ w377 w437 _ _] -> w127
          tunnel: [_ _ w257 _ w374 w433 _ _] -> w126
          tunnel: [_ _ w256 _ w371 w431 _ _] -> w125
          tunnel: [_ _ w255 _ w372 w430 _ _] -> w124
          tunnel: [_ _ w254 _ w373 w432 _ _] -> w123
          tunnel: [_ _ w253 _ w375 w434 _ _] -> w122
          tunnel: [_ _ w252 _ w376 w435 _ _] -> w121
          tunnel: [_ _ w251 _ w370 w436 _ _] -> w120
          tunnel: [_ w195 _ _ _ _ _ w530] -> w118
          tunnel: [_ TRUE _ _ _ _ _ TRUE] -> w119
          frame 0, Default {
            n81 = case shown="0, 默认" w172 {
              tunnel: [FALSE TRUE] -> w175
              tunnel: [w187 w191] -> w157
              tunnel: [_ w190] -> w156
              tunnel: w155 -> [w188 _]
              frame 0, Default {
                n82 = Unbundle By Name(w188) -> ("pH"=w187:u32)
              }
              frame 1 {
                n83 = global read "国弘过程全局变量.vi" "pH"() -> (w192:T7)
                n84 = Unbundle By Name(w192) -> ("命令滤波设定"=w191:u16, "酸碱度偏移修正值"=w190:sgl)
              }
            }
            n85 = in-place {
              n86 = in-place-cluster #4(T5 {"Left"=674, "Top"=256} ("位置 4")) -> ("Top"=w184:i32)
              n87 = in-place-cluster #5(T5 {"Left"=638, "Top"=366} ("位置 7")) -> ("Top"=w180:i32)
              n88 = in-place-cluster #6(T5 {"Left"=674, "Top"=292} ("位置 5")) -> ("Top"=w182:i32)
              n89 = in-place-cluster #7(T5 {"Left"=674, "Top"=221} ("位置 3")) -> ("Top"=w183:i32)
              n90 = in-place-cluster #8(T5 {"Left"=656, "Top"=185} ("位置 2")) -> ("Top"=w185:i32)
              n91 = in-place-cluster #9(T5 {"Left"=674, "Top"=149} ("位置")) -> ("Top"=w186:i32)
              n92 = in-place-cluster #10(T5 {"Left"=710, "Top"=328} ("位置 6")) -> ("Top"=w181:i32)
              n93 = in-place-cluster #4("Top"=w184) -> (w158:T5)
              n94 = in-place-cluster #5("Top"=w180) -> (w167:T5)
              n95 = in-place-cluster #6("Top"=w182) -> (w166:T5)
              n96 = in-place-cluster #7("Top"=w183) -> (w160:T5)
              n97 = in-place-cluster #8("Top"=w185) -> (w162:T5)
              n98 = in-place-cluster #9("Top"=w186) -> (w164:T5)
              n99 = in-place-cluster #10("Top"=w181) -> (w168:T5)
            }
          }
          frame 1 {
            n100 = case shown="0, 默认" w214 {
              tunnel: [FALSE FALSE TRUE] -> w217
              tunnel: [108 ("y") 108 ("y") 72 ("y")] -> w209
              tunnel: w198 -> [w236 w242 _]
              tunnel: [w235 w241 w246] -> w197
              tunnel: [_ _ w247] -> w196
              tunnel: [w233 w239 w245] -> w195
              frame 0, Default {
                n101 = Unbundle By Name(w236) -> ("DO"=w235:u32)
                n102 = global read "禹山过程全局变量.vi" "DO"() -> (w234:cluster{"温度测量值":sgl, "DO%":sgl, "DOmg/L":sgl})
                n103 = Unbundle By Name(w234) -> ("DOmg/L"=w233:sgl)
              }
              frame 2 {
                n104 = Unbundle By Name(w242) -> ("DO"=w241:u32)
                n105 = global read "纳清过程全局变量.vi" "DO测试值"() -> (w240:T8)
                n106 = Unbundle By Name(w240) -> ("溶解氧数值（mg/L）"=w239:sgl)
              }
              frame 1 {
                n107 = global read "国弘过程全局变量.vi" "DO"() -> (w248:T9)
                n108 = Unbundle By Name(w248) -> ("命令滤波设定"=w246:u16, "溶解氧偏移修正值"=w247:sgl, "溶解氧测量值"=w245:sgl)
              }
            }
            n109 = in-place {
              in-place-border: w209 -> [w226]
              n110 = in-place-cluster #11(T5 {"Left"=710, "Top"=328} ("位置 6")) -> ("Top"=w232:i32)
              n111 = in-place-cluster #12(T5 {"Left"=674, "Top"=256} ("位置 4")) -> ("Top"=w223:i32)
              n112 = in-place-cluster #13(T5 {"Left"=638, "Top"=366} ("位置 7")) -> ("Top"=w230:i32)
              n113 = in-place-cluster #14(T5 {"Left"=674, "Top"=292} ("位置 5")) -> ("Top"=w228:i32)
              n114 = in-place-cluster #15(T5 {"Left"=674, "Top"=221} ("位置 3")) -> ("Top"=w222:i32)
              n115 = in-place-cluster #16(T5 {"Left"=656, "Top"=185} ("位置 2")) -> ("Top"=w224:i32)
              n116 = in-place-cluster #17(T5 {"Left"=674, "Top"=149} ("位置")) -> ("Top"=w225:i32)
              n117 = Subtract(x=w230, y=w226) -> (x-y=w229:i32)
              n118 = Subtract(x=w228, y=w226) -> (x-y=w227:i32)
              n119 = Subtract(x=w232, y=w226) -> (x-y=w231:i32)
              n120 = in-place-cluster #11("Top"=w231) -> (w210:T5)
              n121 = in-place-cluster #12("Top"=w223) -> (w199:T5)
              n122 = in-place-cluster #13("Top"=w229) -> (w208:T5)
              n123 = in-place-cluster #14("Top"=w227) -> (w207:T5)
              n124 = in-place-cluster #15("Top"=w222) -> (w201:T5)
              n125 = in-place-cluster #16("Top"=w224) -> (w203:T5)
              n126 = in-place-cluster #17("Top"=w225) -> (w205:T5)
            }
          }
          frame 2 {
            n127 = Unbundle By Name(w261) -> ("Turb"=w260:u32)
            n128 = case shown="2" w280 {
              tunnel: [FALSE TRUE FALSE] -> w283
              tunnel: [0 ("y") 0 ("y") 36 ("y")] -> w275
              tunnel: [_ _ TRUE] -> w264
              tunnel: [_ w303 _] -> w263
              tunnel: [w296 w302 w317] -> w262
              tunnel: w260 -> [w296 _ w317]
              tunnel: [_ _ string[] ["（0-100）NTU", "（0-500）NTU", "（0-2000）NTU", "（0-4000）NTU"]] -> w259
              tunnel: [_ _ w314] -> w258
              tunnel: [_ w301 w312] -> w257
              tunnel: [_ TRUE TRUE] -> w256
              tunnel: [_ _ TRUE] -> w255
              tunnel: [_ _ TRUE] -> w254
              tunnel: [_ _ w309] -> w253
              tunnel: [_ _ w308] -> w252
              tunnel: [_ TRUE TRUE] -> w251
              frame 0, Default {
              }
              frame 1 {
                n129 = global read "国弘过程全局变量.vi" "Turb"() -> (w304:T10)
                n130 = Unbundle By Name(w304) -> ("命令滤波设定"=w302:u16, "浊度偏移修正值"=w303:sgl, "清洁周期"=w301:u16)
              }
              frame 2 {
                n131 = global read "纳清过程全局变量.vi" "浊度测试值"() -> (w315:T11)
                n132 = Unbundle By Name(w315) -> ("清扫模式"=w308:u16, "清扫次数"=w309:u16, "清扫间隔分钟"=w312:u16, "量程"=w314:u16)
              }
            }
            n133 = in-place {
              in-place-border: w275 -> [w287]
              n134 = in-place-cluster #18(T5 {"Left"=674, "Top"=256} ("位置 4")) -> ("Top"=w293:i32)
              n135 = in-place-cluster #19(T5 {"Left"=638, "Top"=366} ("位置 7")) -> ("Top"=w290:i32)
              n136 = in-place-cluster #20(T5 {"Left"=674, "Top"=292} ("位置 5")) -> ("Top"=w291:i32)
              n137 = in-place-cluster #21(T5 {"Left"=674, "Top"=221} ("位置 3")) -> ("Top"=w292:i32)
              n138 = in-place-cluster #22(T5 {"Left"=656, "Top"=185} ("位置 2")) -> ("Top"=w294:i32)
              n139 = in-place-cluster #23(T5 {"Left"=674, "Top"=149} ("位置")) -> ("Top"=w295:i32)
              n140 = in-place-cluster #24(T5 {"Left"=710, "Top"=328} ("位置 6")) -> ("Top"=w289:i32)
              n141 = Subtract(x=w292, y=w287) -> (x-y=w288:i32)
              n142 = in-place-cluster #18("Top"=w293) -> (w265:T5)
              n143 = in-place-cluster #19("Top"=w290) -> (w274:T5)
              n144 = in-place-cluster #20("Top"=w291) -> (w273:T5)
              n145 = in-place-cluster #21("Top"=w288) -> (w267:T5)
              n146 = in-place-cluster #22("Top"=w294) -> (w269:T5)
              n147 = in-place-cluster #23("Top"=w295) -> (w271:T5)
              n148 = in-place-cluster #24("Top"=w289) -> (w276:T5)
            }
          }
          frame 3 {
            n149 = Unbundle By Name(w324) -> ("Cond"=w323:u32)
            n150 = case shown="2" w342 {
              tunnel: [FALSE TRUE FALSE] -> w345
              tunnel: [0 ("y") 36 ("y") 72 ("y")] -> w337
              tunnel: [_ TRUE TRUE] -> w325
              tunnel: w323 -> [w357 _ w366]
              tunnel: [w357 w360 w366] -> w322
              tunnel: [_ w361 _] -> w321
              frame 0, Default {
              }
              frame 1 {
                n151 = global read "国弘过程全局变量.vi" "Cond"() -> (w362:T12)
                n152 = Unbundle By Name(w362) -> ("命令滤波设定"=w360:u16, "电导率偏移修正值"=w361:sgl)
              }
              frame 2 {
              }
            }
            n153 = in-place {
              in-place-border: w337 -> [w349]
              n154 = in-place-cluster #25(T5 {"Left"=674, "Top"=256} ("位置 4")) -> ("Top"=w354:i32)
              n155 = in-place-cluster #26(T5 {"Left"=638, "Top"=366} ("位置 7")) -> ("Top"=w352:i32)
              n156 = in-place-cluster #27(T5 {"Left"=710, "Top"=328} ("位置 6")) -> ("Top"=w351:i32)
              n157 = in-place-cluster #28(T5 {"Left"=674, "Top"=292} ("位置 5")) -> ("Top"=w353:i32)
              n158 = in-place-cluster #29(T5 {"Left"=674, "Top"=221} ("位置 3")) -> ("Top"=w348:i32)
              n159 = in-place-cluster #30(T5 {"Left"=656, "Top"=185} ("位置 2")) -> ("Top"=w355:i32)
              n160 = in-place-cluster #31(T5 {"Left"=674, "Top"=149} ("位置")) -> ("Top"=w356:i32)
              n161 = Subtract(x=w354, y=w349) -> (x-y=w350:i32)
              n162 = in-place-cluster #25("Top"=w350) -> (w327:T5)
              n163 = in-place-cluster #26("Top"=w352) -> (w336:T5)
              n164 = in-place-cluster #27("Top"=w351) -> (w338:T5)
              n165 = in-place-cluster #28("Top"=w353) -> (w335:T5)
              n166 = in-place-cluster #29("Top"=w348) -> (w329:T5)
              n167 = in-place-cluster #30("Top"=w355) -> (w331:T5)
              n168 = in-place-cluster #31("Top"=w356) -> (w333:T5)
            }
          }
          frame 4 {
            n169 = case shown="2" w397 {
              tunnel: [FALSE TRUE FALSE] -> w400
              tunnel: [0 ("y") 0 ("y") 36 ("y")] -> w392
              tunnel: [_ _ TRUE] -> w381
              tunnel: [_ _ string[] ["（0-500）μg/L", "（0-50）μg/L"]] -> w378
              tunnel: [_ _ w424] -> w377
              tunnel: [_ _ w423] -> w376
              tunnel: [_ _ w422] -> w375
              tunnel: [_ _ w421] -> w374
              tunnel: [_ _ TRUE] -> w373
              tunnel: [_ _ TRUE] -> w372
              tunnel: [_ _ TRUE] -> w371
              tunnel: [_ _ TRUE] -> w370
              frame 0, Default {
              }
              frame 1 {
              }
              frame 2 {
                n170 = global read "纳清过程全局变量.vi" "叶绿素a测试值"() -> (w425:T13)
                n171 = Unbundle By Name(w425) -> ("量程"=w424:u16, "清扫模式"=w423:u16, "清扫次数"=w422:u16, "清扫间隔分钟"=w421:u16)
              }
            }
            n172 = Unbundle By Name(w380) -> ("叶绿素a"=w379:u32)
            n173 = in-place {
              in-place-border: w392 -> [w404]
              n174 = in-place-cluster #32(T5 {"Left"=674, "Top"=221} ("位置 3")) -> ("Top"=w409:i32)
              n175 = in-place-cluster #33(T5 {"Left"=656, "Top"=185} ("位置 2")) -> ("Top"=w411:i32)
              n176 = in-place-cluster #34(T5 {"Left"=674, "Top"=256} ("位置 4")) -> ("Top"=w410:i32)
              n177 = in-place-cluster #35(T5 {"Left"=638, "Top"=366} ("位置 7")) -> ("Top"=w407:i32)
              n178 = in-place-cluster #36(T5 {"Left"=674, "Top"=292} ("位置 5")) -> ("Top"=w408:i32)
              n179 = in-place-cluster #37(T5 {"Left"=710, "Top"=328} ("位置 6")) -> ("Top"=w406:i32)
              n180 = in-place-cluster #38(T5 {"Left"=674, "Top"=149} ("位置")) -> ("Top"=w412:i32)
              n181 = Subtract(x=w409, y=w404) -> (x-y=w405:i32)
              n182 = in-place-cluster #32("Top"=w405) -> (w384:T5)
              n183 = in-place-cluster #33("Top"=w411) -> (w386:T5)
              n184 = in-place-cluster #34("Top"=w410) -> (w382:T5)
              n185 = in-place-cluster #35("Top"=w407) -> (w391:T5)
              n186 = in-place-cluster #36("Top"=w408) -> (w390:T5)
              n187 = in-place-cluster #37("Top"=w406) -> (w393:T5)
              n188 = in-place-cluster #38("Top"=w412) -> (w388:T5)
            }
          }
          frame 5 {
            n189 = case shown="2" w457 {
              tunnel: [FALSE TRUE FALSE] -> w460
              tunnel: [0 ("y") 0 ("y") 36 ("y")] -> w452
              tunnel: [_ _ TRUE] -> w441
              tunnel: [_ _ string[] ["（0-2000000）c/mL", "（0-200000）c/mL"]] -> w438
              tunnel: [_ _ w484] -> w437
              tunnel: [_ _ TRUE] -> w436
              tunnel: [_ _ w482] -> w435
              tunnel: [_ _ w481] -> w434
              tunnel: [_ _ w480] -> w433
              tunnel: [_ _ TRUE] -> w432
              tunnel: [_ _ TRUE] -> w431
              tunnel: [_ _ TRUE] -> w430
              frame 0, Default {
              }
              frame 1 {
              }
              frame 2 {
                n190 = global read "纳清过程全局变量.vi" "蓝绿藻测试值"() -> (w485:T14)
                n191 = Unbundle By Name(w485) -> ("量程"=w484:u16, "清扫模式"=w482:u16, "清扫次数"=w481:u16, "清扫间隔分钟"=w480:u16)
              }
            }
            n192 = Unbundle By Name(w440) -> ("藻密度"=w439:u32)
            n193 = in-place {
              in-place-border: w452 -> [w464]
              n194 = in-place-cluster #39(T5 {"Left"=674, "Top"=221} ("位置 3")) -> ("Top"=w469:i32)
              n195 = in-place-cluster #40(T5 {"Left"=656, "Top"=185} ("位置 2")) -> ("Top"=w471:i32)
              n196 = in-place-cluster #41(T5 {"Left"=674, "Top"=256} ("位置 4")) -> ("Top"=w470:i32)
              n197 = in-place-cluster #42(T5 {"Left"=638, "Top"=366} ("位置 7")) -> ("Top"=w467:i32)
              n198 = in-place-cluster #43(T5 {"Left"=674, "Top"=292} ("位置 5")) -> ("Top"=w468:i32)
              n199 = in-place-cluster #44(T5 {"Left"=710, "Top"=328} ("位置 6")) -> ("Top"=w466:i32)
              n200 = in-place-cluster #45(T5 {"Left"=674, "Top"=149} ("位置")) -> ("Top"=w472:i32)
              n201 = Subtract(x=w469, y=w464) -> (x-y=w465:i32)
              n202 = in-place-cluster #39("Top"=w465) -> (w444:T5)
              n203 = in-place-cluster #40("Top"=w471) -> (w446:T5)
              n204 = in-place-cluster #41("Top"=w470) -> (w442:T5)
              n205 = in-place-cluster #42("Top"=w467) -> (w451:T5)
              n206 = in-place-cluster #43("Top"=w468) -> (w450:T5)
              n207 = in-place-cluster #44("Top"=w466) -> (w453:T5)
              n208 = in-place-cluster #45("Top"=w472) -> (w448:T5)
            }
          }
          frame 6 {
            n209 = Unbundle By Name(w491) -> ("ORP"=w490:u32)
            n210 = case shown="0, 默认" w508 {
              tunnel: [FALSE TRUE] -> w511
              tunnel: [_ w526] -> w493
              tunnel: [w523 w525] -> w492
              tunnel: w490 -> [w523 _]
              frame 0, Default {
              }
              frame 1 {
                n211 = global read "国弘过程全局变量.vi" "ORP"() -> (w527:T15)
                n212 = Unbundle By Name(w527) -> ("命令滤波设定"=w525:u16, "偏移修正值"=w526:sgl)
              }
            }
            n213 = in-place {
              n214 = in-place-cluster #46(T5 {"Left"=710, "Top"=328} ("位置 6")) -> ("Top"=w517:i32)
              n215 = in-place-cluster #47(T5 {"Left"=674, "Top"=256} ("位置 4")) -> ("Top"=w520:i32)
              n216 = in-place-cluster #48(T5 {"Left"=638, "Top"=366} ("位置 7")) -> ("Top"=w516:i32)
              n217 = in-place-cluster #49(T5 {"Left"=674, "Top"=292} ("位置 5")) -> ("Top"=w518:i32)
              n218 = in-place-cluster #50(T5 {"Left"=674, "Top"=221} ("位置 3")) -> ("Top"=w519:i32)
              n219 = in-place-cluster #51(T5 {"Left"=656, "Top"=185} ("位置 2")) -> ("Top"=w521:i32)
              n220 = in-place-cluster #52(T5 {"Left"=674, "Top"=149} ("位置")) -> ("Top"=w522:i32)
              n221 = in-place-cluster #46("Top"=w517) -> (w504:T5)
              n222 = in-place-cluster #47("Top"=w520) -> (w494:T5)
              n223 = in-place-cluster #48("Top"=w516) -> (w503:T5)
              n224 = in-place-cluster #49("Top"=w518) -> (w502:T5)
              n225 = in-place-cluster #50("Top"=w519) -> (w496:T5)
              n226 = in-place-cluster #51("Top"=w521) -> (w498:T5)
              n227 = in-place-cluster #52("Top"=w522) -> (w500:T5)
            }
          }
          frame 7 {
            n228 = case shown="0, 默认" w549 {
              tunnel: [FALSE TRUE] -> w552
              tunnel: [108 ("y") 72 ("y")] -> w544
              frame 0, Default {
              }
              frame 1 {
              }
            }
            n229 = Unbundle By Name(w533) -> ("DO"=w532:u32)
            n230 = global read "禹山过程全局变量.vi" "DO 2"() -> (w531:cluster{"温度测量值":sgl, "DO%":sgl, "DOmg/L":sgl})
            n231 = Unbundle By Name(w531) -> ("DOmg/L"=w530:sgl)
            n232 = in-place {
              in-place-border: w544 -> [w561]
              n233 = in-place-cluster #53(T5 {"Left"=638, "Top"=366} ("位置 7")) -> ("Top"=w565:i32)
              n234 = in-place-cluster #54(T5 {"Left"=674, "Top"=292} ("位置 5")) -> ("Top"=w563:i32)
              n235 = in-place-cluster #55(T5 {"Left"=710, "Top"=328} ("位置 6")) -> ("Top"=w567:i32)
              n236 = in-place-cluster #56(T5 {"Left"=674, "Top"=256} ("位置 4")) -> ("Top"=w558:i32)
              n237 = in-place-cluster #57(T5 {"Left"=674, "Top"=221} ("位置 3")) -> ("Top"=w557:i32)
              n238 = in-place-cluster #58(T5 {"Left"=656, "Top"=185} ("位置 2")) -> ("Top"=w559:i32)
              n239 = in-place-cluster #59(T5 {"Left"=674, "Top"=149} ("位置")) -> ("Top"=w560:i32)
              n240 = Subtract(x=w565, y=w561) -> (x-y=w564:i32)
              n241 = Subtract(x=w563, y=w561) -> (x-y=w562:i32)
              n242 = Subtract(x=w567, y=w561) -> (x-y=w566:i32)
              n243 = in-place-cluster #53("Top"=w564) -> (w543:T5)
              n244 = in-place-cluster #54("Top"=w562) -> (w542:T5)
              n245 = in-place-cluster #55("Top"=w566) -> (w545:T5)
              n246 = in-place-cluster #56("Top"=w558) -> (w534:T5)
              n247 = in-place-cluster #57("Top"=w557) -> (w536:T5)
              n248 = in-place-cluster #58("Top"=w559) -> (w538:T5)
              n249 = in-place-cluster #59("Top"=w560) -> (w540:T5)
            }
          }
        }
        n250 = property on="恢复出厂" class="Bool"("Visible"=w116) -> ()  [unwired: 2 in, 2 out]
        n251 = property on="校准温度" class="Bool"("DisabledEnum"=w115) -> ()  [unwired: 2 in, 2 out]
        n252 = global read "断电保存变量.vi" "盐度自动获取"() -> (w132:bool)
        n253 = property on="清洗选板" class="TabCtl (严格)"("Visible"=w120) -> ()  [unwired: 2 in, 2 out]
        n254 = property on="清扫模式" class="Ring (严格)"("Visible"=w123, "Value"=w121) -> ()  [unwired: 2 in, 2 out]
        n255 = property on="溶解氧浓度值" class="DigNum (严格)"("Visible"=w119, "Value"=w118) -> ()  [unwired: 2 in, 2 out]
        n256 = property on="温度系数" class="DigNum (严格)"("Position"=w144, "Visible"=w137) -> ()  [unwired: 2 in, 2 out]
        n257 = property on="测量量程" class="Ring (严格)"("Position"=w145, "Visible"=w139, "Strings []"=w128, "Value"=w127) -> ()  [unwired: 2 in, 2 out]
        n258 = property on="清扫间隔" class="DigNum (严格)"("Visible"=w125, "Value"=w126) -> ()  [unwired: 2 in, 2 out]
        n259 = property on="盐度" class="DigNum (严格)"("Position"=w142, "Visible"=w138) -> ()  [unwired: 2 in, 2 out]
        n260 = property on="偏移修正值" class="DigNum (严格)"("Position"=w146, "Visible"=w136, "Value"=w130) -> ()  [unwired: 2 in, 2 out]
        n261 = property on="滤波次数" class="DigNum (严格)"("Position"=w148, "Visible"=w140, "Value"=w131) -> ()  [unwired: 2 in, 2 out]
        n262 = property on="清扫次数" class="DigNum (严格)"("Visible"=w124, "Value"=w122) -> ()  [unwired: 2 in, 2 out]
        n263 = global read "断电保存变量.vi" "大气压补偿"() -> (w133:dbl)
        n264 = property on="自动盐度补偿" class="Bool (严格)"("Position"=w141, "Visible"=w135, "Value"=w132) -> ()  [unwired: 2 in, 2 out]
        n265 = property on="大气压力" class="DigNum (严格)"("Position"=w143, "Visible"=w134, "Value"=w133) -> ()  [unwired: 2 in, 2 out]
      }
    }
    n266 = Wait (ms)(milliseconds to wait=u32 1000 ("等待时间（毫秒）")) -> ()  [unwired: 1 out]
  }
  n267 = while {
    tunnel: w1 -> [w574]
    stop <- FALSE stop-if-true
    n268 = Wait on Occurrence(2:w574) -> (0:w572:bool)  [unwired: 2 in]
    n269 = flat-sequence {
      tunnel: w572 -> [_]
      frame #0 {
        n270 = call "信号曲线.vi"() -> ()  [unwired: 12 in]
      }
    }
  }
  n271 = property on="窗格" class="Pane"("Origin"=T1 {"Horizontal"=0, "Vertical"=0} ("原点")) -> ()  [unwired: 2 in, 2 out]
  n272 = while {
    tunnel: w1 -> [w575]
    stop <- FALSE stop-if-true
    n273 = event shown="[12] \"标液一.标准值\", \"标液二.标准值\", \"标液三.标准值\", \"实际温度\", \"大气压力\", \"盐度\", \"滤波次数\", \"偏移修正值\", \"温度系数\", \"标液一.原始值\", \"标液三.原始值\", \"标液二.原始值\": 鼠标按下" {
      selector: _ -> [_ _ _ _ _ _ _ _ _ _ _ _ _ _ _ _ _ _ _]
      dyn-events: _ -> [_ _ _ _ _ _ _ _ _ _ _ _ _ _ _ _ _ _ _]
      timeout: _ -> [_ _ _ _ _ _ _ _ _ _ _ _ _ _ _ _ _ _ _]
      tunnel: w575 -> [_ w577 _ _ _ _ _ _ _ _ _ _ _ _ _ _ _ _ _]
      event Timeout {
        n274 = event-data() -> ()  [unwired: 1 in, 3 out]
      }
      event "显示曲线": Value Change {
        n275 = event-data() -> ()  [unwired: 1 in, 6 out]
        n276 = Set Occurrence(w577) -> ()
      }
      event "温度系数": Value Change {
        n277 = event-data() -> ()  [unwired: 1 in, 6 out]
        n278 = property on="校准参数" class="Ring (严格)"() -> ("Value"=w581:u16)  [unwired: 2 in, 2 out]
        n279 = call "探头温度系数.vi"("校准参数"=w581, "温度系数"="温度系数") -> ("error out"=w578:errorcluster)  [unwired: 9 in]
        n280 = case shown="错误" w578 {
          tunnel: ["设置成功！" "设置失败！"] -> w579
          frame No Error {
          }
          frame Error {
          }
        }
        n281 = One Button Dialog(message=w579) -> ()  [unwired: 1 in, 1 out]
      }
      event "恢复出厂": Value Change {
        n282 = event-data() -> ()  [unwired: 1 in, 6 out]
        n283 = property on="校准参数" class="Ring (严格)"() -> ("Value"=w586:u16)  [unwired: 2 in, 2 out]
        n284 = call "探头恢复出厂.vi"("校准参数"=w586) -> ("error out"=w584:errorcluster)  [unwired: 10 in]
        n285 = case shown="错误" w584 {
          tunnel: ["设置成功！" "设置失败！"] -> w585
          frame No Error {
          }
          frame Error {
          }
        }
        n286 = One Button Dialog(message=w585) -> ()  [unwired: 1 in, 1 out]
      }
      event "测量量程": Value Change {
        n287 = event-data() -> ()  [unwired: 1 in, 6 out]
        n288 = property on="校准参数" class="Ring (严格)"() -> ("Value"=w591:u16)  [unwired: 2 in, 2 out]
        n289 = call "探头校准量程设置.vi"("校准参数"=w591, "校准量程"="测量量程") -> ("error out"=w590:errorcluster)  [unwired: 9 in]
        n290 = call "探头测量量程设置.vi"("校准参数"=w591, "error in (no error)"=w590, "测量量程设置"="测量量程") -> ("error out"=w592:errorcluster)  [unwired: 8 in]
        n291 = case shown="错误" w592 {
          tunnel: ["设置成功！" "设置失败！"] -> w593
          frame No Error {
          }
          frame Error {
          }
        }
        n292 = One Button Dialog(message=w593) -> ()  [unwired: 1 in, 1 out]
      }
      event "自动盐度补偿", "大气压力", "盐度", "滤波次数": Value Change {
        n293 = event-data() -> ()  [unwired: 1 in, 6 out]
        n294 = flat-sequence {
          tunnel: [w597] -> w596
          tunnel: w596 -> [_]
          frame #0 {
            n295 = property on="校准参数" class="Ring (严格)"() -> ("Value"=w599:u16)  [unwired: 2 in, 2 out]
            n296 = global write "断电保存变量.vi" "大气压补偿"("大气压力") -> ()
            n297 = call "探头滤波次数.vi"("校准参数"=w599, "滤波次数"="滤波次数") -> ("error out"=w597:errorcluster)  [unwired: 9 in]
            n298 = global write "断电保存变量.vi" "盐度自动获取"("自动盐度补偿") -> ()
            n299 = global write "断电保存变量.vi" "盐度补偿"("盐度") -> ()
          }
          frame #1 {
            n300 = call "配置文件保存.vi"() -> ()  [unwired: 12 in]
          }
        }
      }
      event "清洗": Value Change {
        n301 = event-data() -> ()  [unwired: 1 in, 6 out]
        n302 = property on="校准参数" class="Ring (严格)"() -> ("Value"=w603:u16)  [unwired: 2 in, 2 out]
        n303 = call "探头手动清洗.vi"("校准参数"=w603) -> ("error out"=w604:errorcluster)  [unwired: 10 in]
        n304 = case shown="无错误" w604 {
          tunnel: ["启动成功！" "启动失败！"] -> w605
          frame No Error {
          }
          frame Error {
          }
        }
        n305 = One Button Dialog(message=w605) -> ()  [unwired: 1 in, 1 out]
      }
      event "清扫模式": Value Change {
        n306 = event-data() -> ()  [unwired: 1 in, 6 out]
        n307 = property on="校准参数" class="Ring (严格)"() -> ("Value"=w609:u16)  [unwired: 2 in, 2 out]
        n308 = case shown="5" w609 {
          tunnel: [T16."null" ("探头") T16."pH" ("探头") T16."DO" ("探头") T16."浊度" ("探头") T16."电导率" ("探头") T16."叶绿素a" ("探头") T16."藻密度" ("探头")] -> w608
          frame Default {
          }
          frame 0 {
          }
          frame 1 {
          }
          frame 2 {
          }
          frame 3 {
          }
          frame 4 {
          }
          frame 5 {
          }
        }
        n309 = call "纳清_清扫模式.vi"("探头"=w608, "清扫模式"="清扫模式") -> ("error out"=w610:errorcluster)  [unwired: 9 in]
        n310 = case shown="错误" w610 {
          tunnel: ["设置成功！" "设置失败！"] -> w611
          frame No Error {
          }
          frame Error {
          }
        }
        n311 = One Button Dialog(message=w611) -> ()  [unwired: 1 in, 1 out]
      }
      event "清扫次数": Value Change {
        n312 = event-data() -> ()  [unwired: 1 in, 6 out]
        n313 = property on="校准参数" class="Ring (严格)"() -> ("Value"=w626:u16)  [unwired: 2 in, 2 out]
        n314 = case shown="5" w626 {
          tunnel: [T16."null" ("探头") T16."pH" ("探头") T16."DO" ("探头") T16."浊度" ("探头") T16."电导率" ("探头") T16."叶绿素a" ("探头") T16."藻密度" ("探头")] -> w625
          frame Default {
          }
          frame 0 {
          }
          frame 1 {
          }
          frame 2 {
          }
          frame 3 {
          }
          frame 4 {
          }
          frame 5 {
          }
        }
        n315 = call "纳清_清扫次数.vi"("探头"=w625, "清扫次数"="清扫次数") -> ("error out"=w623:errorcluster)  [unwired: 9 in]
        n316 = case shown="错误" w623 {
          tunnel: ["设置成功！" "设置失败！"] -> w624
          frame No Error {
          }
          frame Error {
          }
        }
        n317 = One Button Dialog(message=w624) -> ()  [unwired: 1 in, 1 out]
      }
      event "清扫间隔": Value Change {
        n318 = event-data() -> ()  [unwired: 1 in, 6 out]
        n319 = property on="校准参数" class="Ring (严格)"() -> ("Value"=w637:u16)  [unwired: 2 in, 2 out]
        n320 = call "探头清洗间隔.vi"("校准参数"=w637, "清扫间隔"="清扫间隔") -> ("error out"=w636:errorcluster)  [unwired: 9 in]
        n321 = case shown="错误" w636 {
          tunnel: ["设置成功！" "设置失败！"] -> w639
          frame No Error {
          }
          frame Error {
          }
        }
        n322 = One Button Dialog(message=w639) -> ()  [unwired: 1 in, 1 out]
      }
      event "校准温度": Value Change {
        n323 = event-data() -> ()  [unwired: 1 in, 6 out]
        n324 = property on="校准参数" class="Ring (严格)"() -> ("Value"=w645:u16)  [unwired: 2 in, 2 out]
        n325 = call "温度校准.vi"("校准参数"=w645, "校准温度"="实际温度") -> ("error out"=w644:errorcluster)  [unwired: 9 in]
        n326 = case shown="错误" w644 {
          tunnel: ["校准成功！" "校准失败！"] -> w643
          frame No Error {
          }
          frame Error {
          }
        }
        n327 = One Button Dialog(message=w643) -> ()  [unwired: 1 in, 1 out]
      }
      event "偏移修正值": Value Change {
        n328 = event-data() -> ()  [unwired: 1 in, 6 out]
        n329 = property on="校准参数" class="Ring (严格)"() -> ("Value"=w649:u16)  [unwired: 2 in, 2 out]
        n330 = call "探头偏移修正值.vi"("校准参数"=w649, "温度偏移修正值"="偏移修正值") -> ("error out"=w650:errorcluster)  [unwired: 9 in]
        n331 = case shown="无错误" w650 {
          tunnel: ["设置成功！" "设置失败！"] -> w651
          frame No Error {
          }
          frame Error {
          }
        }
        n332 = One Button Dialog(message=w651) -> ()  [unwired: 1 in, 1 out]
      }
      event "标液一.标准值", "标液二.标准值", "标液三.标准值", "实际温度", "大气压力", "盐度", "滤波次数", "偏移修正值", "温度系数", "标液一.原始值", "标液三.原始值", "标液二.原始值": Mouse Down {
        n333 = event-data() -> ("CtlRef"=w657:refnum<vi>)  [unwired: 1 in, 7 out]
        n334 = property class="DigNum (严格)"(reference=w657) -> (reference out=w655:refnum<vi>, "Value"=w656:dbl)  [unwired: 1 in, 1 out]
        n335 = call "数字键盘.vi"("OldNumber"=w656) -> ("NewNumber"=w654:dbl)  [unwired: 1 in]
        n336 = property class="DigNum (严格)"(reference=w655, "Val(Sgnl)"=w654) -> ()  [unwired: 1 in, 2 out]
      }
      event "清扫次数", "清扫间隔": Mouse Down {
        n337 = event-data() -> ("CtlRef"=w661:refnum<vi>)  [unwired: 1 in, 7 out]
        n338 = property class="DigNum (严格)"(reference=w661) -> (reference out=w659:refnum<vi>, "Value"=w660:u16)  [unwired: 1 in, 1 out]
        n339 = call "数字键盘.vi"("OldNumber"=w660) -> ("NewNumber"=w658:dbl)  [unwired: 1 in]
        n340 = property class="DigNum (严格)"(reference=w659, "Val(Sgnl)"=w658) -> ()  [unwired: 1 in, 2 out]
      }
      event "标液一.标准值", "标液二.标准值", "标液三.标准值": Value Change {
        n341 = event-data() -> ()  [unwired: 1 in, 6 out]
        n342 = property on="校准参数" class="Ring (严格)"() -> ("Value"=w665:u16)  [unwired: 2 in, 2 out]
        n343 = property on="标准值" class="DigNum (严格)"() -> ("Value"=w664:dbl)  [unwired: 2 in, 2 out]
        n344 = property on="标准值" class="DigNum (严格)"() -> ("Value"=w663:dbl)  [unwired: 2 in, 2 out]
        n345 = property on="标准值" class="DigNum (严格)"() -> ("Value"=w662:dbl)  [unwired: 2 in, 2 out]
        n346 = call "探头校准标准值设置.vi"("校准参数"=w665, "标液三"=w662, "标液二"=w663, "标液一"=w664) -> ()  [unwired: 8 in]
      }
      event "校准参数": Value Change {
        n347 = event-data() -> ()  [unwired: 1 in, 6 out]
        n348 = property on="校准参数" class="Ring (严格)"() -> ("Value"=w668:u16)  [unwired: 2 in, 2 out]
        n349 = call "探头型号.vi"("校准参数"=w668) -> ("禁用项[]"=w667:i32[], "value"=w666:i32)  [unwired: 8 in, 1 out]
        n350 = property on="校准方式" class="Ring (严格)"("Disabled Items []"=w667, "Val(Sgnl)"=w666) -> ()  [unwired: 2 in, 2 out]
      }
      event "校准方式": Value Change {
        n351 = event-data() -> ()  [unwired: 1 in, 6 out]
        n352 = property on="校准参数" class="Ring (严格)"() -> ("Value"=w671:u16)  [unwired: 2 in, 2 out]
        n353 = call "探头型号.vi"("校准参数"=w671) -> ("探头型号"=w670:u16)  [unwired: 8 in, 2 out]
        n354 = case shown="1" w670 {
          tunnel: [_ TRUE] -> w669
          frame 0, Default {
          }
          frame 1 {
          }
        }
        n355 = flat-sequence {
          tunnel: w669 -> [w673]
          frame #0 {
            n356 = property on="校准方式" class="Ring (严格)"() -> ("Value"=w672:u16)  [unwired: 2 in, 2 out]
            n357 = case shown="1" w672 {
              tunnel: [cluster{bool, bool, bool} {TRUE, FALSE, FALSE} cluster{bool, bool, bool} {TRUE, TRUE, FALSE} cluster{bool, bool, bool} {TRUE, TRUE, TRUE}] -> w679
              frame 0, Default {
              }
              frame 1 {
              }
              frame 2 {
              }
            }
            n358 = Unbundle(w679) -> (w678:bool, w676:bool, w677:bool)
            n359 = property on="标液一开始校准" class="Bool (严格)"("Visible"=w678) -> ()  [unwired: 2 in, 2 out]
            n360 = property on="第一点确认校准" class="Bool"("Visible"=w678) -> ()  [unwired: 2 in, 2 out]
            n361 = property on="标液一" class="Clust (严格)"("Visible"=w678) -> ()  [unwired: 2 in, 2 out]
            n362 = property on="标液二开始校准" class="Bool (严格)"("Visible"=w676) -> ()  [unwired: 2 in, 2 out]
            n363 = property on="标液二" class="Clust (严格)"("Visible"=w676) -> ()  [unwired: 2 in, 2 out]
            n364 = property on="标液三" class="Clust (严格)"("Visible"=w677) -> ()  [unwired: 2 in, 2 out]
            n365 = property on="标液三开始校准" class="Bool (严格)"("Visible"=w677) -> ()  [unwired: 2 in, 2 out]
            n366 = And(x=w673, y=w676) -> (x .and. y?=w675:bool)
            n367 = And(x=w677, y=w673) -> (x .and. y?=w674:bool)
            n368 = property on="第二点确认校准" class="Bool"("Visible"=w675) -> ()  [unwired: 2 in, 2 out]
            n369 = property on="第三点确认校准" class="Bool"("Visible"=w674) -> ()  [unwired: 2 in, 2 out]
          }
        }
      }
      event "标液一开始校准", "标液二开始校准", "标液三开始校准": Value Change {
        n370 = event-data() -> ("CtlRef"=w696:refnum<vi>, "NewVal"=w684:bool)  [unwired: 1 in, 4 out]
        n371 = Select(t=T4."Disabled and Grayed Out" ("禁用 3"), s=w684, f=T4."Enabled") -> (s? t:f=w686:T4)
        n372 = property class="Bool (严格)"(reference=w696) -> ("Label.Text"=w695:string)  [unwired: 1 in, 2 out]
        n373 = case shown="假" w684 {
          tunnel: [_ w698] -> w685
          frame False {
          }
          frame True {
            n374 = property on="校准参数" class="Ring (严格)"() -> ("Value"=w697:u16)  [unwired: 2 in, 2 out]
            n375 = case shown="4" w697 {
              tunnel: [T2 {"ph"=TRUE, "DO"=FALSE, "Cond"=FALSE, "Turb"=FALSE, "叶绿素a"=FALSE, "藻密度"=FALSE, "ORP"=FALSE, "COD"=FALSE, "DO2"=FALSE} ("校准运行状态") T2 {"ph"=FALSE, "DO"=TRUE, "Cond"=FALSE, "Turb"=FALSE, "叶绿素a"=FALSE, "藻密度"=FALSE, "ORP"=FALSE, "COD"=FALSE, "DO2"=FALSE} ("校准运行状态") T2 {"ph"=FALSE, "DO"=FALSE, "Cond"=FALSE, "Turb"=TRUE, "叶绿素a"=FALSE, "藻密度"=FALSE, "ORP"=FALSE, "COD"=FALSE, "DO2"=FALSE} ("校准运行状态") T2 {"ph"=FALSE, "DO"=FALSE, "Cond"=TRUE, "Turb"=FALSE, "叶绿素a"=FALSE, "藻密度"=FALSE, "ORP"=FALSE, "COD"=FALSE, "DO2"=FALSE} ("校准运行状态") T2 {"ph"=FALSE, "DO"=FALSE, "Cond"=FALSE, "Turb"=FALSE, "叶绿素a"=TRUE, "藻密度"=FALSE, "ORP"=FALSE, "COD"=FALSE, "DO2"=FALSE} ("校准运行状态") T2 {"ph"=FALSE, "DO"=FALSE, "Cond"=FALSE, "Turb"=FALSE, "叶绿素a"=FALSE, "藻密度"=TRUE, "ORP"=FALSE, "COD"=FALSE, "DO2"=FALSE} ("校准运行状态") T2 {"ph"=FALSE, "DO"=FALSE, "Cond"=FALSE, "Turb"=FALSE, "叶绿素a"=FALSE, "藻密度"=FALSE, "ORP"=TRUE, "COD"=FALSE, "DO2"=FALSE} ("校准运行状态") T2 {"ph"=FALSE, "DO"=FALSE, "Cond"=FALSE, "Turb"=FALSE, "叶绿素a"=FALSE, "藻密度"=FALSE, "ORP"=FALSE, "COD"=FALSE, "DO2"=TRUE} ("校准运行状态")] -> w698
              frame 0, Default {
              }
              frame 1 {
              }
              frame 2 {
              }
              frame 3 {
              }
              frame 4 {
              }
              frame 5 {
              }
              frame 6 {
              }
              frame 7 {
              }
            }
          }
        }
        n376 = case shown="\"标液三开始校准\"" w695 {
          tunnel: [w708 w710 w712] -> _
          tunnel: [T17 {"禁用"=enum."Enabled", "禁用 2"=enum."Disabled and Grayed Out", "禁用 3"=enum."Disabled and Grayed Out"} T17 {"禁用"=enum."Disabled and Grayed Out", "禁用 2"=enum."Enabled", "禁用 3"=enum."Disabled and Grayed Out"} T17 {"禁用"=enum."Disabled and Grayed Out", "禁用 2"=enum."Disabled and Grayed Out", "禁用 3"=enum."Enabled"}] -> w693
          frame "标液一开始校准", Default {
            w708 = u16 0 items=["第一点", "第二点", "第三点"] ("当前校准点位")
          }
          frame "标液二开始校准" {
            w710 = u16 1 items=["第一点", "第二点", "第三点"] ("当前校准点位")
          }
          frame "标液三开始校准" {
            w712 = u16 2 items=["第一点", "第二点", "第三点"] ("当前校准点位")
          }
        }
        n377 = property on="校准参数" class="Ring (严格)"("DisabledEnum"=w686) -> ()  [unwired: 2 in, 2 out]
        n378 = property on="校准方式" class="Ring (严格)"("DisabledEnum"=w686) -> ()  [unwired: 2 in, 2 out]
        n379 = property on="第二点确认校准" class="Bool"("DisabledEnum"=w686) -> ()  [unwired: 2 in, 2 out]
        n380 = property on="第三点确认校准" class="Bool"("DisabledEnum"=w686) -> ()  [unwired: 2 in, 2 out]
        n381 = property on="第一点确认校准" class="Bool"("DisabledEnum"=w686) -> ()  [unwired: 2 in, 2 out]
        n382 = Select(t=w693, s=w684, f=T17 {"禁用"=enum."Enabled", "禁用 2"=enum."Enabled", "禁用 3"=enum."Enabled"}) -> (s? t:f=w692:T17)
        n383 = Unbundle(w692) -> ("禁用"=w694:T4, "禁用 2"=w688:T4, "禁用 3"=w687:T4)
        n384 = global write "多参数全局变量.vi" "校准运行状态"(w685) -> ()
        n385 = property on="标液一开始校准" class="Bool (严格)"("DisabledEnum"=w694) -> ()  [unwired: 2 in, 2 out]
        n386 = property on="标液二开始校准" class="Bool (严格)"("DisabledEnum"=w688) -> ()  [unwired: 2 in, 2 out]
        n387 = property on="标液三开始校准" class="Bool (严格)"("DisabledEnum"=w687) -> ()  [unwired: 2 in, 2 out]
      }
      event "第一点确认校准", "第二点确认校准", "第三点确认校准": Value Change {
        n388 = event-data() -> ("CtlRef"=w727:refnum<vi>)  [unwired: 1 in, 5 out]
        n389 = property on="校准参数" class="Ring (严格)"() -> ("Value"=w722:u16)  [unwired: 2 in, 2 out]
        n390 = call "探头型号.vi"("校准参数"=w722) -> ("探头型号"=w728:u16)  [unwired: 8 in, 2 out]
        n391 = property on="校准方式" class="Ring (严格)"() -> ("Value"=w719:u16)  [unwired: 2 in, 2 out]
        n392 = property on="校准参数" class="Ring (严格)"() -> ("Value"=w720:u16)  [unwired: 2 in, 2 out]
        n393 = case shown="1" w728 {
          tunnel: [w755 w767] -> w716
          tunnel: w727 -> [_ w770]
          tunnel: [TRUE w757] -> w721
          tunnel: w719 -> [_ w768]
          tunnel: w720 -> [_ _]
          tunnel: [errorcluster {"status"=FALSE, "code"=0, "source"="校准成功！"} ("error in (no error)") w759] -> w715
          tunnel: [errorcluster {"status"=TRUE, "code"=0, "source"="校准失败！"} ("error in (no error)") w758] -> w714
          frame 0, Default {
            n394 = property on="校准方式" class="Ring (严格)"() -> ("Value"=w755:u16)  [unwired: 2 in, 2 out]
          }
          frame 1 {
            n395 = property class="Bool"(reference=w770) -> ("Label.Text"=w769:string)  [unwired: 1 in, 2 out]
            n396 = case shown="\"第一点确认校准\", 默认" w769 {
              tunnel: [u16 0 ("Value") u16 1 ("Value") u16 2 ("Value")] -> w767
              tunnel: ["第一点校准通过，请更换标液，准备第二点校准！" "第二点校准通过，请更换标液，准备第三点校准！" "校准成功！"] -> w766
              tunnel: ["第一点校准失败，请重新校准！" "第二点校准失败，请重新校准！" "第三点校准失败，请重新校准！"] -> w764
              frame "第一点确认校准", Default {
              }
              frame "第二点确认校准" {
              }
              frame "第三点确认校准" {
              }
            }
            n397 = Equal?(x=w768, y=w767) -> (x = y?=w757:bool)
            n398 = Select(t="校准成功！", s=w757, f=w766) -> (s? t:f=w762:string)
            n399 = Select(t="校准失败！", s=w757, f=w764) -> (s? t:f=w761:string)
            n400 = Bundle By Name(cluster=errorcluster {"status"=FALSE, "code"=0, "source"="校准成功！"} ("error in (no error)"), "source"=w762) -> (w759:errorcluster)
            n401 = Bundle By Name(cluster=errorcluster {"status"=TRUE, "code"=0, "source"="校准失败！"} ("error in (no error)"), "source"=w761) -> (w758:errorcluster)
          }
        }
        n402 = property on="标液一" class="Clust (严格)"() -> ("Value"=w725:cluster{"标准值":dbl, "检测值":dbl, "原始值":dbl})  [unwired: 2 in, 2 out]
        n403 = property on="标液二" class="Clust (严格)"() -> ("Value"=w724:cluster{"标准值":dbl, "检测值":dbl, "原始值":dbl})  [unwired: 2 in, 2 out]
        n404 = property on="标液三" class="Clust (严格)"() -> ("Value"=w723:cluster{"标准值":dbl, "检测值":dbl, "原始值":dbl})  [unwired: 2 in, 2 out]
        n405 = property on="测量量程" class="Ring (严格)"() -> ("Value"=w713:u16)  [unwired: 2 in, 2 out]
        n406 = call "执行校准.vi"("校准点位"=w716, "校准方式"=w719, "校准量程"=w713, "校准参数"=w720, "标液三"=w723, "标液二"=w724, "标液一"=w725) -> ("error out"=w718:errorcluster)  [unwired: 4 in]
        n407 = case shown="无错误" w718 {
          selector: w718 -> [_ w750]
          tunnel: [w743 "校准失败！"] -> w726
          tunnel: [w744 w750] -> w717
          tunnel: w715 -> [w742 _]
          tunnel: w714 -> [w741 _]
          frame No Error {
            n408 = flat-sequence {
              tunnel: [w747] -> w745
              frame #0 {
                n409 = Wait (ms)(milliseconds to wait=u32 2000 ("等待时间（毫秒）")) -> ()  [unwired: 1 out]
              }
              frame #1 {
                n410 = property on="电极状态标志" class="DigNum (严格)"() -> ("Value"=w748:u16)  [unwired: 2 in, 2 out]
                n411 = case shown="默认" w748 {
                  tunnel: [_ TRUE] -> w747
                  frame Default {
                  }
                  frame 0..2, 31..33 {
                  }
                }
              }
            }
            n412 = Select(t=w742, s=w745, f=w741) -> (s? t:f=w744:errorcluster)
            n413 = Unbundle By Name(w744) -> ("source"=w743:string)
          }
          frame Error {
          }
        }
        n414 = One Button Dialog(message=w726) -> ()  [unwired: 1 in, 1 out]
        n415 = case shown="真" w721 {
          tunnel: w725 -> [_ w740]
          tunnel: w724 -> [_ w739]
          tunnel: w723 -> [_ w738]
          tunnel: w720 -> [_ w729]
          tunnel: w719 -> [_ w733]
          tunnel: w717 -> [_ w737]
          frame False {
          }
          frame True {
            n416 = call "探头测量值显示.vi"("校准参数"=w729) -> ("线性系数"=w732:cluster{bool, "K":sgl, "B":sgl})  [unwired: 3 in, 7 out]
            n417 = Unbundle By Name(w732) -> ("K"=w731:sgl, "B"=w730:sgl)
            n418 = control-ref of="校准记录"() -> (w735:refnum<vi>)
            n419 = property on="当前温度" class="DigNum (严格)"() -> ("Value"=w736:dbl)  [unwired: 2 in, 2 out]
            n420 = property on="序列号" class="Str"() -> ("Value"=w734:string)  [unwired: 2 in, 2 out]
            n421 = call "生成校准记录.vi"("标液一"=w740, "校准参数"=w729, "校准方式"=w733, "校准记录"=w735, "标液二"=w739, "标液三"=w738, "当前温度"=w736, "error in (no error)"=w737, "序列号"=w734, "K"=w731, "B"=w730) -> ()  [unwired: 3 in, 2 out]
          }
        }
      }
    }
  }
  n422 = while {
    shift-right: [w783] -> _
    shift-left: _ -> [w782]
    shift-left: _ -> [w781]
    stop <- FALSE stop-if-true
    n423 = Not Equal?(x=w782, y=w781) -> (x != y?=w780:bool)
    n424 = case shown="真" w780 {
      frame False {
      }
      frame True {
        n425 = global write "多参数全局变量.vi" "重新获取KB值命令"(TRUE ("重新获取KB值命令")) -> ()
      }
    }
    n426 = Wait (ms)(milliseconds to wait=u32 1000 ("等待时间（毫秒）")) -> ()  [unwired: 1 out]
    n427 = global read "多参数全局变量.vi" "当前页面"() -> (w784:enum16{"主页面", "参数页面", "校准页面"})
    n428 = global read "多参数全局变量.vi" "校准参数"() -> (w785:u16)
    n429 = Add(x=w784, y=w785) -> (x+y=w783:u16)
  }
